vi "P2019 TB INCAR_Run Auto.vi"(7 "ModuloIN":u32=10, 8 "error in (no error)":errorcluster, 9 "Comunicaciones":T7={"Flujo_1"="ASRL6::INSTR", "Brk1"=FALSE, "Flujo_2"="ASRL6::INSTR", "Brk2"=FALSE, "Flujo_3"="ASRL6::INSTR", "Brk3"=FALSE, "Flujo_4"="ASRL6::INSTR", "Brk4"=FALSE, "Eurothe"="ASRL6::INSTR", "Eurot"=FALSE, "Balanza"="ASRL6::INSTR", "Bal"=FALSE, "eValPos"="ASRL6::INSTR", "eVal"=FALSE, "flowbus"="ASRL6::INSTR", "fb"=FALSE}, 10 "Secuencia":string[](array[string])) -> (0 "error out":errorcluster)   [LabVIEW 2013]
uses:
  Controles/P2022 Datos Control.ctl
  Controles/P2018 Com Control.ctl
  modbusEurotherm P116_485/4xP116.ctl
  Controles/P2018 DisbalTB Control.ctl
  Controles/P2018 Arduino Control.ctl
  Controles/P2018 Bronkhorst Control.ctl
  serialBronkhorst/_s_TablaBronkhorst.ctl
  modbusEurotherm P116_485/P2018 Eurotherm Control.ctl
  Controles/Data Type.ctl
  Display/Display_Command Control.ctl
  Controles/P2018 runAuto Control.ctl
  File/File_Module Control.ctl
  Timing/Timing_Module Control.ctl
  modbusEurotherm P116_485/Eurotherm_Hardware_Module Control.ctl
  serialTermobDisbal/Multicard III_Hardware_Module Control.ctl
  P2022 TB INCAR GLOBALES.vi
panel:
  out "Valvula":bool=TRUE
  out "TIEMPO (m)":dbl
  out "EURO_P116":T1
  out "BRONKHORST":T3={"Dispositivos"=[["3", "NO", "M0000013", "Air", "10", "ln/mn", "0", "0"], ["4", "NO", "M0000014", "Air", "10", "ln/mn", "0", "0"], ["5", "NO", "M0000015", "Air", "10", "ln/mn", "0", "0"], ["6", "NO", "M0000016", "Air", "10", "ln/mn", "0", "0"], ["7", "NO", "M0000017", "Air", "10", "ln/mn", "0", "0"], ["8", "NO", "M0000018", "Air", "10", "ln/mn", "0", "0"]], "NuevosSP"=[["0", "NO", "M0000013", "Air", "1", "ln/mn", "0", "0"], ["0", "NO", "M0000014", "Air", "1", "ln/mn", "0", "0"], ["0", "NO", "M0000015", "Air", "1", "ln/mn", "0", "0"], ["0", "NO", "M0000016", "Air", "1", "ln/mn", "0", "0"], ["0", "NO", "M0000017", "Air", "1", "ln/mn", "0", "0"], ["0", "NO", "M0000018", "Air", "1", "ln/mn", "0", "0"]], "Nodes"=8, "Delay(s)"=0.075}
  out "ARDUINO":T5
  out "DISBAL":T6 caption="tarjetaPresion"
  out "RateSP":T2
  out "NuevoSP":T2
  out "Modulo":u32
  out "Timestring":string
  out "MedidaModulo":u32
  out "Max_t(s)":dbl format="%.1f"
  out "Delta t(s)":dbl format="%.1f"
  out "Delta T(C)":dbl format="%.1f"
  out "TStable":bool
  out "Datos":T8 {"fFSET4" format="%.2g"; "fFSET3" format="%.2g"; "fFSET2" format="%.2g"; "fFSET1" format="%.2g"; "fFLUJO4" format="%.2g"; "fFLUJO2" format="%.2g"; "fFLUJO1" format="%.2g"; "fFLUJO3" format="%.2g"; "T_EXTRA" format="%.2g"; "TSET_EXTRA" format="%.2g"; "T_CINTA" format="%.2g"; "TSET_CINTA" format="%.2g"; "sFSET4" format="%.2g"; "POSICION" format="%.2g"; "TEMP_SUP" format="%.2g"; "TSET_SUP" format="%.2g"; "PESO_TB" format="%.2g"; "TEMP_TB" format="%.2g"; "TEMP_INF" format="%.2g"; "sFSET3" format="%.2g"; "sFSET2" format="%.2g"; "sFSET1" format="%.2g"; "V_VAPOR" format="%.2g"; "sFLUJO4" format="%.2g"; "sFLUJO2" format="%.2g"; "sFLUJO1" format="%.2g"; "TSET_INF" format="%.2g"; "TIEMPO" format="%.2g"; "sFLUJO3" format="%.2g"}
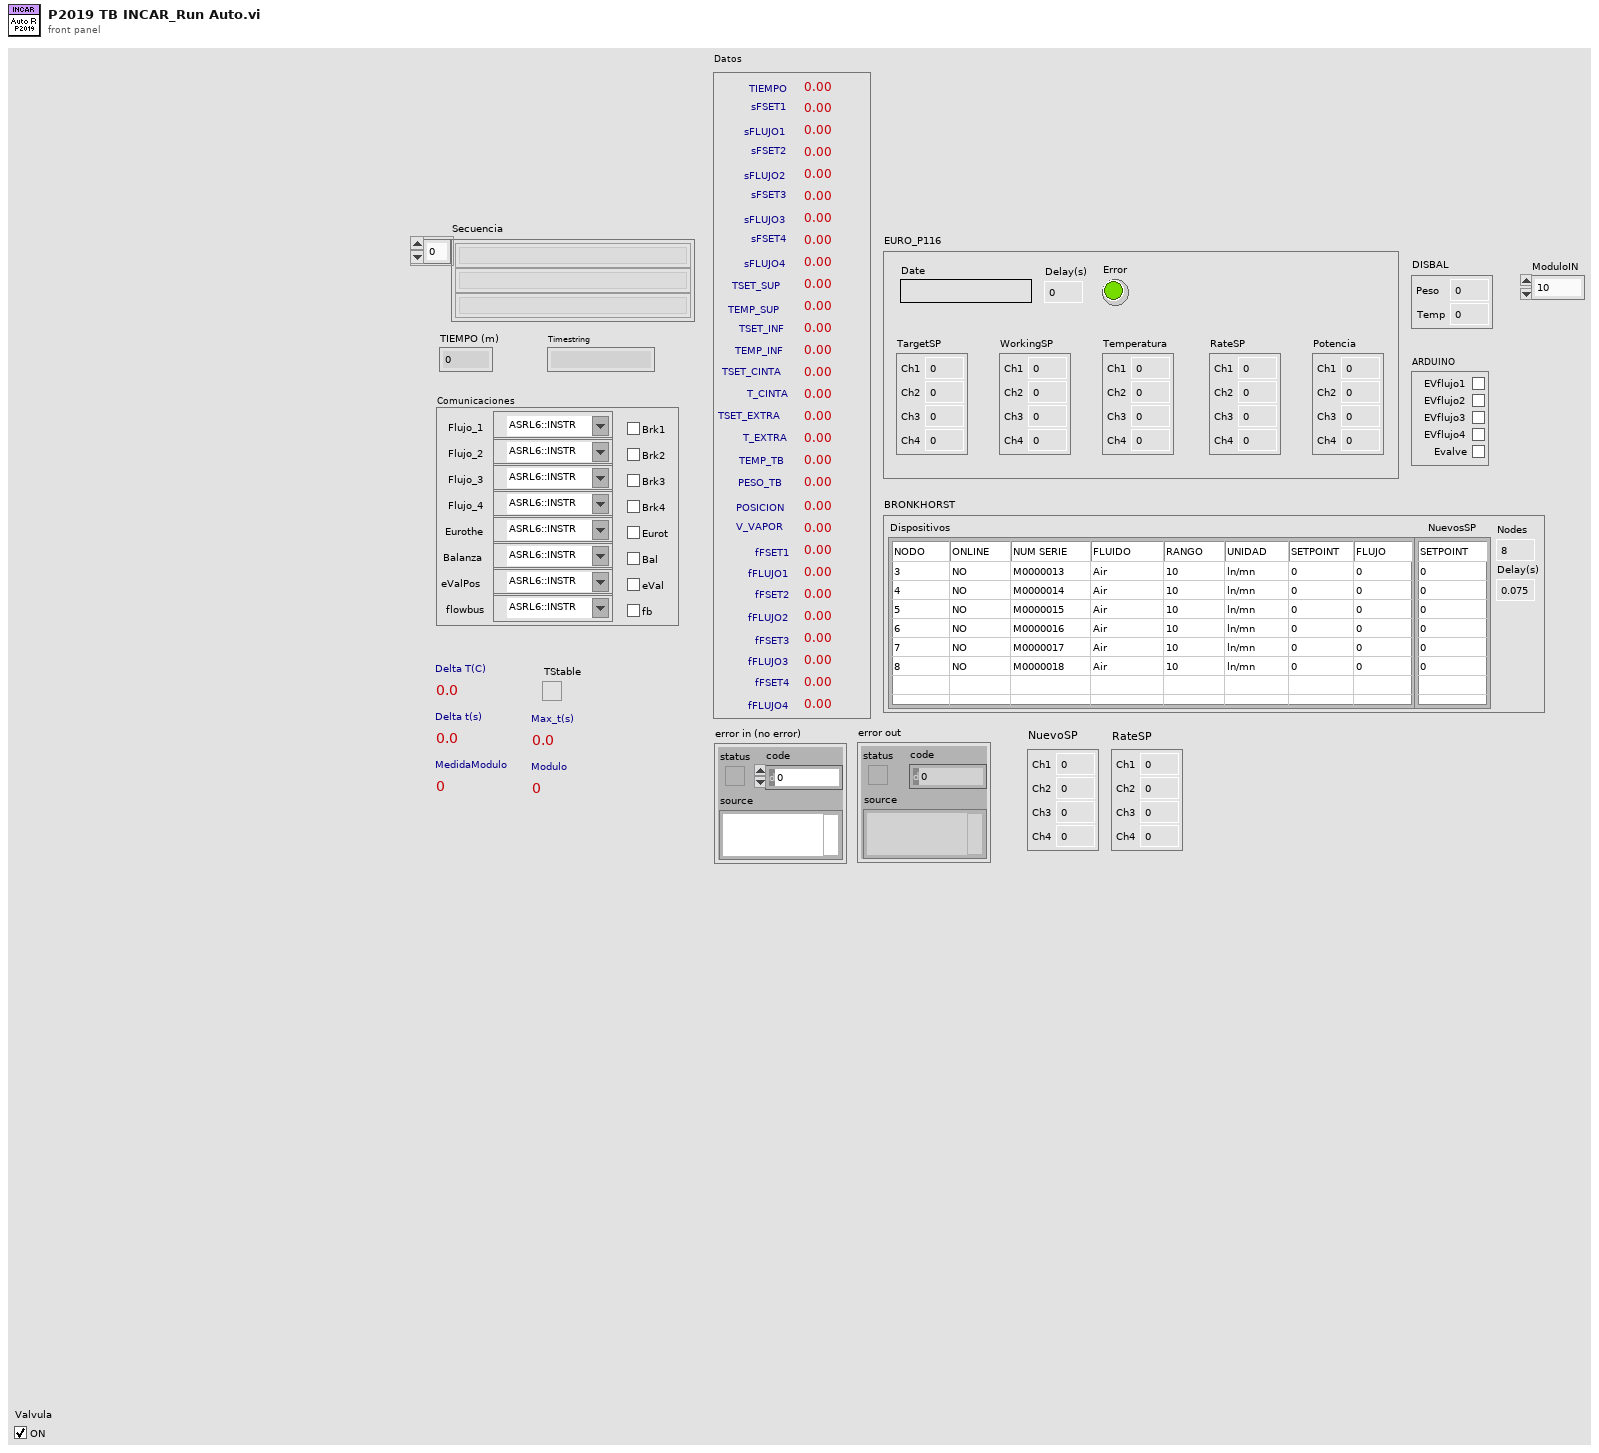
[diagram p1: front panel]
types:
  T1 = typedef "P2018 Eurotherm Control.ctl" = cluster{"TargetSP":T2, "WorkingSP":T2, "Temperatura":T2, "Error":bool, "Date":string, "Delay(s)":dbl, "RateSP":T2, "Potencia":T2}
  T2 = typedef "4xP116.ctl" = cluster{"Ch1":dbl, "Ch2":dbl, "Ch3":dbl, "Ch4":dbl}
  T3 = typedef "P2018 Bronkhorst Control.ctl" = cluster{"Dispositivos":T4, "NuevosSP":string[][], "Nodes":u32, "Delay(s)":dbl}
  T4 = typedef "_s_TablaBronkhorst.ctl" = string[][]
  T5 = typedef "P2018 Arduino Control.ctl" = cluster{"EVflujo1":bool, "EVflujo2":bool, "EVflujo3":bool, "EVflujo4":bool, "Evalve":bool}
  T6 = typedef "P2018 DisbalTB Control.ctl" = cluster{"Peso":dbl, "Temp":dbl}
  T7 = typedef "P2018 Com Control.ctl" = cluster{"Flujo_1":refnum<visa-resource-name>, "Brk1":bool, "Flujo_2":refnum<visa-resource-name>, "Brk2":bool, "Flujo_3":refnum<visa-resource-name>, "Brk3":bool, "Flujo_4":refnum<visa-resource-name>, "Brk4":bool, "Eurothe":refnum<visa-resource-name>, "Eurot":bool, "Balanza":refnum<visa-resource-name>, "Bal":bool, "eValPos":refnum<visa-resource-name>, "eVal":bool, "flowbus":refnum<visa-resource-name>, "fb":bool}
  T8 = typedef "P2022 Datos Control.ctl" = cluster{"TIEMPO":dbl, "sFSET1":dbl, "sFLUJO1":dbl, "sFSET2":dbl, "sFLUJO2":dbl, "sFSET3":dbl, "sFLUJO3":dbl, "sFSET4":dbl, "sFLUJO4":dbl, "TSET_SUP":dbl, "TEMP_SUP":dbl, "TSET_INF":dbl, "TEMP_INF":dbl, "TSET_CINTA":dbl, "T_CINTA":dbl, "TSET_EXTRA":dbl, "T_EXTRA":dbl, "TEMP_TB":dbl, "PESO_TB":dbl, "POSICION":dbl, "V_VAPOR":dbl, "fFSET1":dbl, "fFLUJO1":dbl, "fFSET2":dbl, "fFLUJO2":dbl, "fFSET3":dbl, "fFLUJO3":dbl, "fFSET4":dbl, "fFLUJO4":dbl}
  T9 = typedef "Data Type.ctl" = enum16{"Init FP", "En/Dis FP Ctls", "Update FP", "Upd Status", "Upd Seq"}
  T10 = typedef "Display_Command Control.ctl" = enum16{"Initialize", "Generate Event", "Shutdown"}
  T11 = typedef "P2018 runAuto Control.ctl" = enum16{"inicializar", "testComando", "cambioGasesS", "cambioGasesF", "cambioValvulas", "cambioTemperaturas", "cEstableTemp?", "cReadTiempo", "cReadGases", "cReadTemperaturas", "cReadTermobalanza", "cSaveDatos", "cWait", "cambioTiempos", "tAgotadoTiempo?", "tReadTiempo", "tReadGases", "tReadTemperaturas", "tReadTermobalanza", "tSaveDatos", "tWait", "finalizar"}
  T12 = typedef "File_Module Control.ctl" = enum16{"Initialize", "Save Head", "Save Data", "Shutdown"}
  T13 = typedef "Eurotherm_Hardware_Module Control.ctl" = enum16{"Initialize", "Write SP", "Read SP+PV", "Write Rate", "Set P", "Set I", "Set D", "Shutdown"}
  T14 = typedef "Timing_Module Control.ctl" = enum16{"Initialize Time", "Check Time"}
  T15 = typedef "Multicard III_Hardware_Module Control.ctl" = enum16{"Initialize", "Cero", "Span", "Read ugr", "Read mgr", "Read A/D", "Read T", "Number readings", "Thermocouple type", "Status", "Shutdown"}
  T16 = typedef "P2019 SetpointsFlows.ctl" = cluster{"SP1":dbl, "SP2":dbl, "SP3":dbl, "SP4":dbl}
  T17 = typedef "_f_TablaBronkhorst.ctl" = string[][]
  T18 = enum16{"Add 1", "Add 2", "Add 10", "Add 11", "Add 12", "Add 13"}[]
  T19 = cluster{"processVal":dbl, "targetSP":dbl, "workingSP":dbl, "workingOut":dbl}
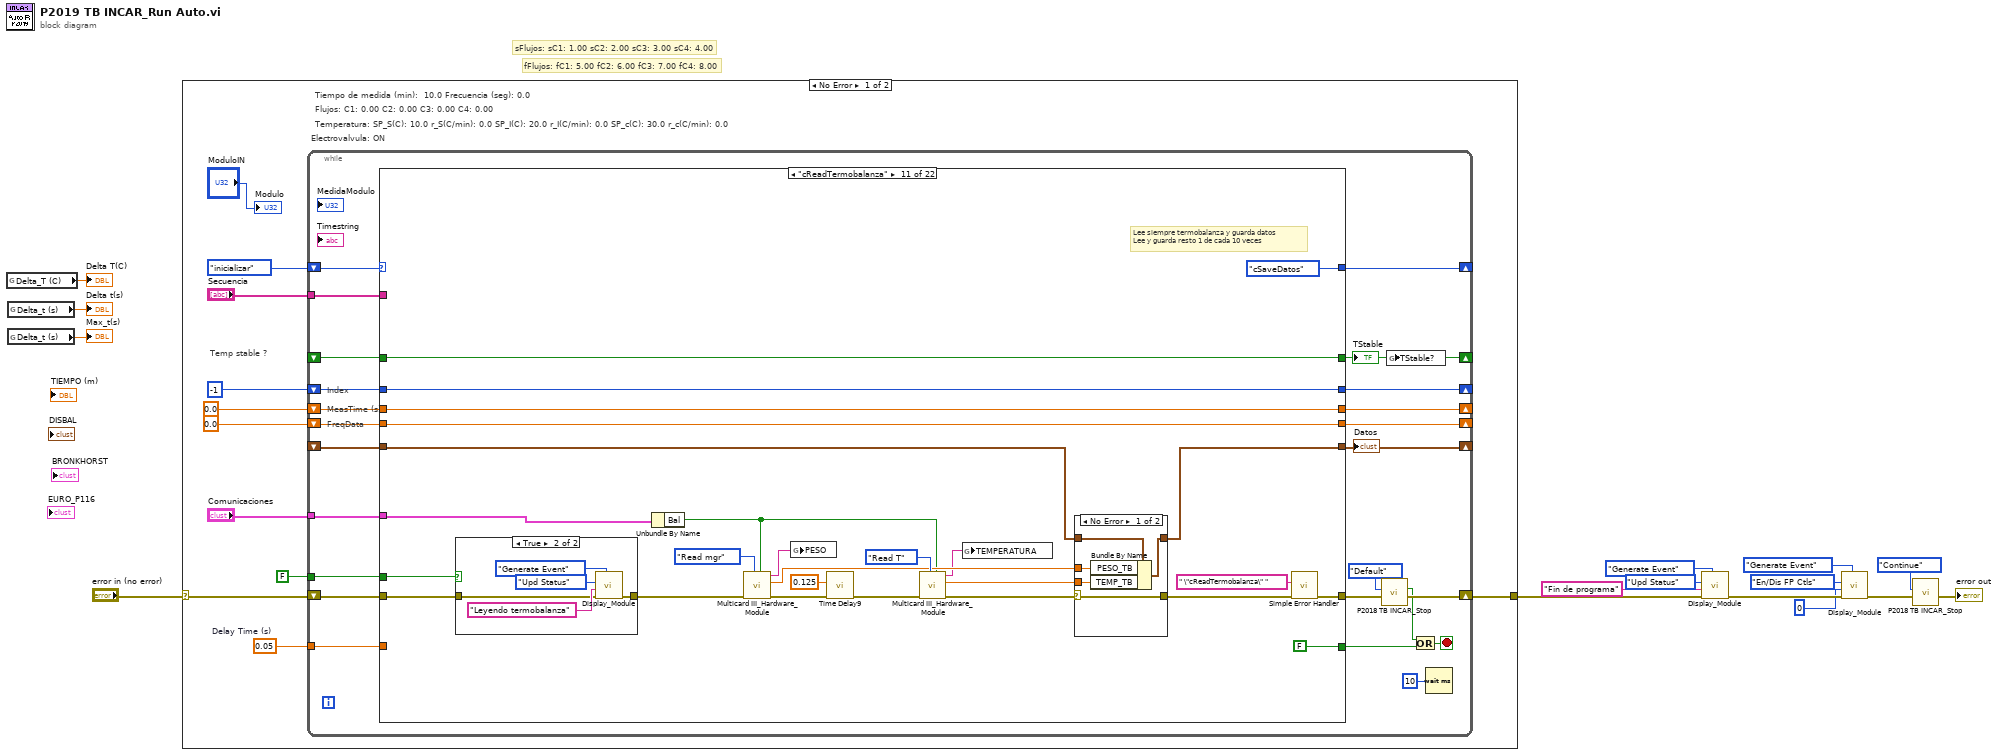
[diagram p0: block diagram]
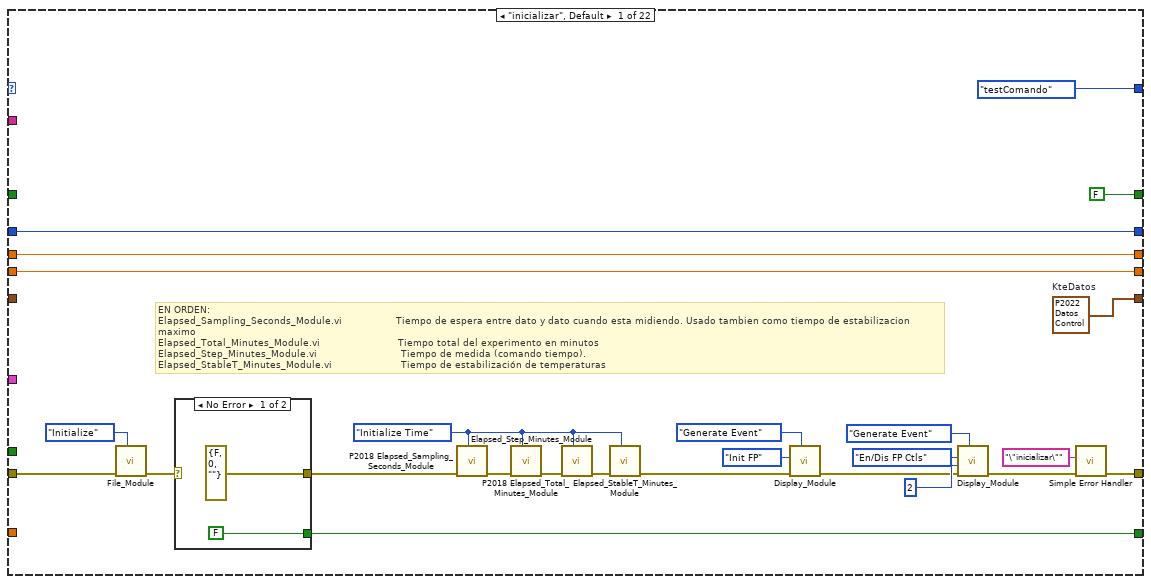
[diagram p2: hidden frame]
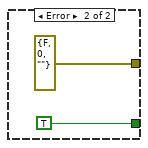
[diagram p3: hidden frame]
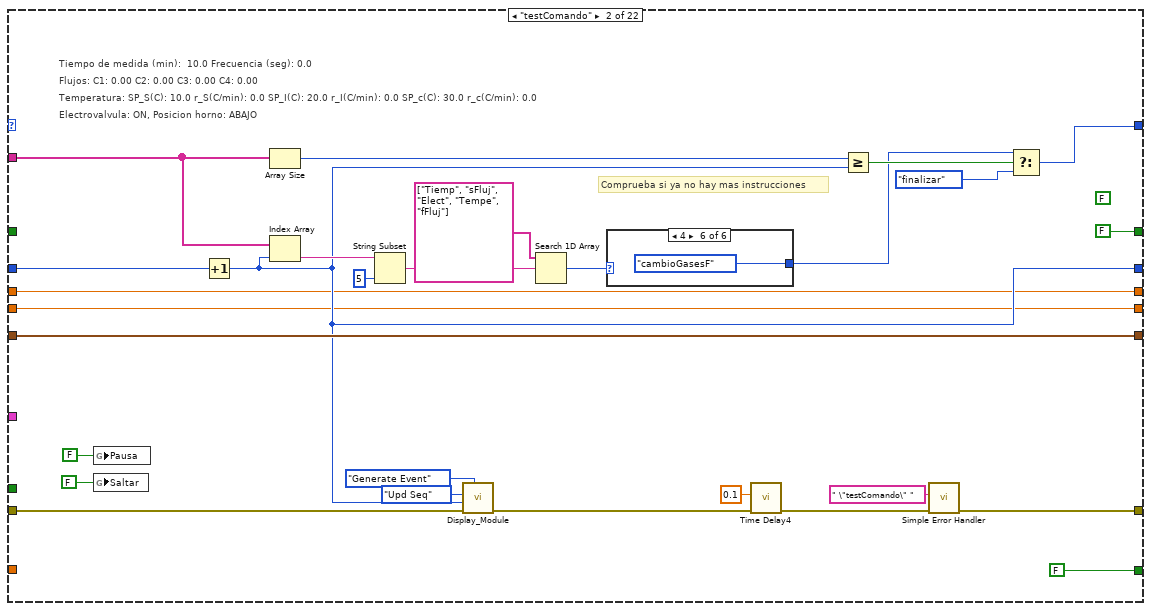
[diagram p4: hidden frame]
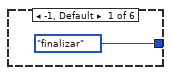
[diagram p5: hidden frame]
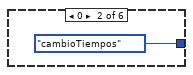
[diagram p6: hidden frame]
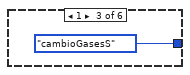
[diagram p7: hidden frame]
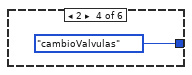
[diagram p8: hidden frame]
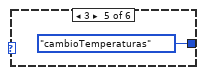
[diagram p9: hidden frame]
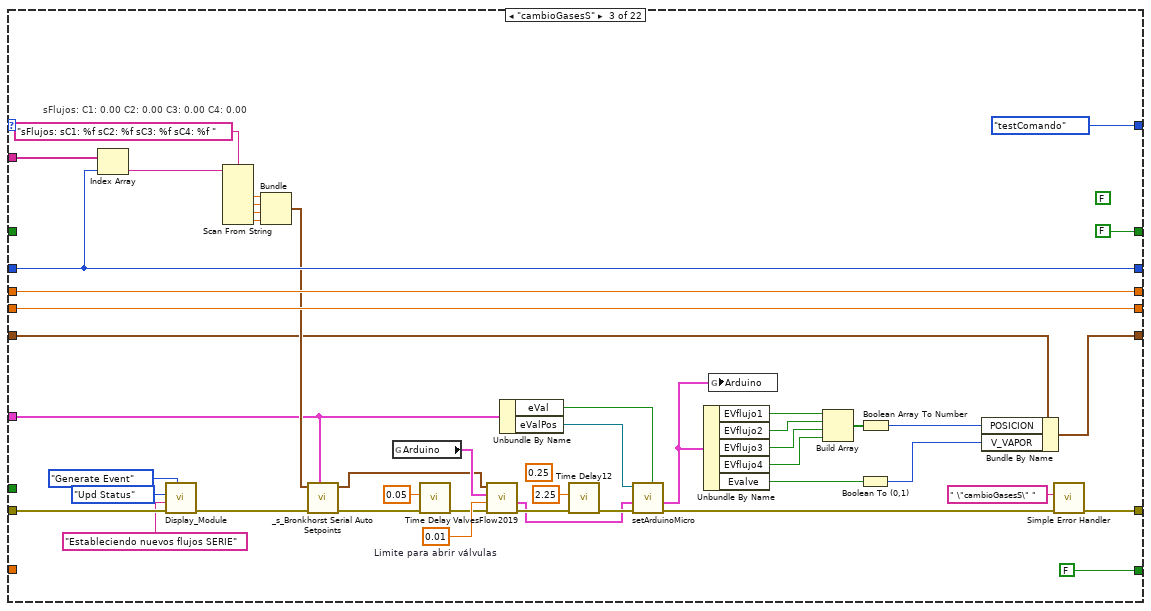
[diagram p10: hidden frame]
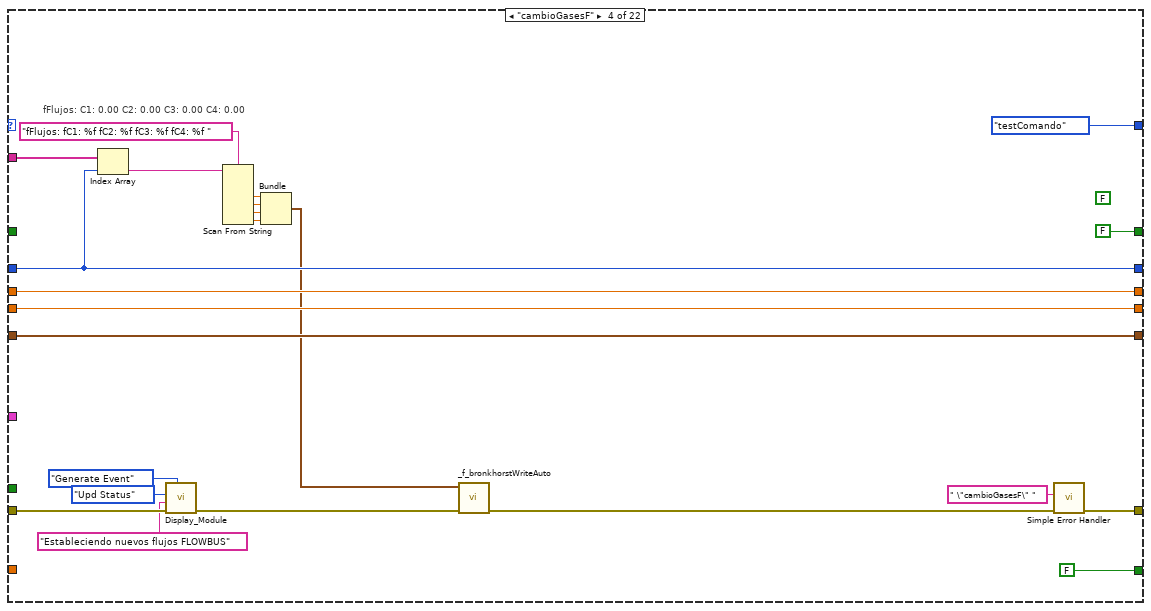
[diagram p11: hidden frame]
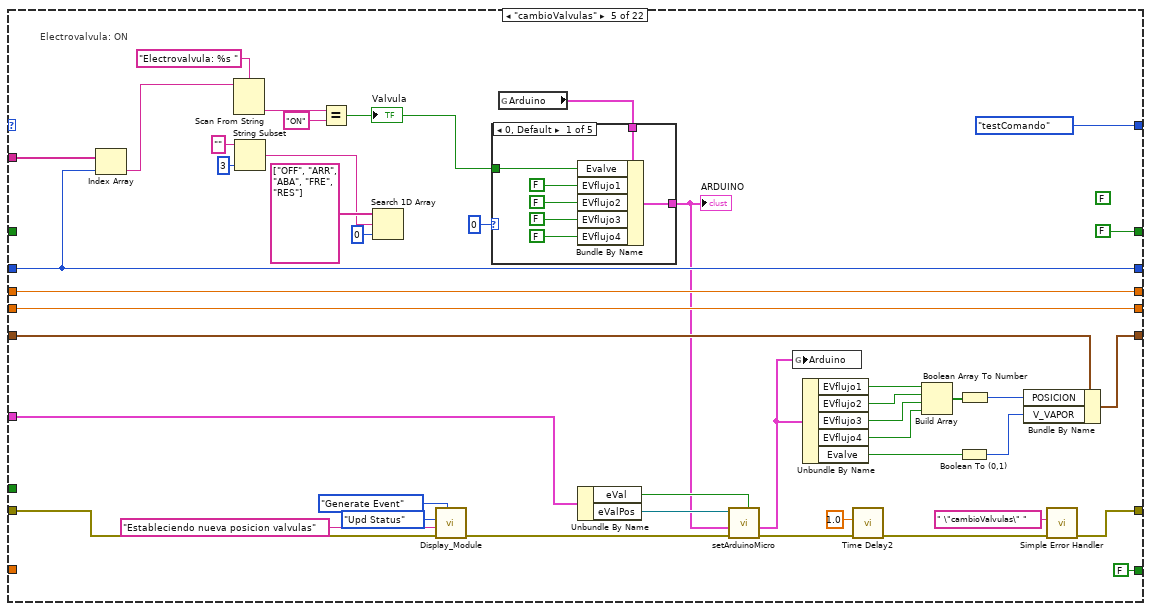
[diagram p12: hidden frame]
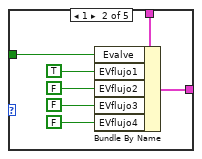
[diagram p13: hidden frame]
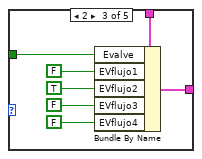
[diagram p14: hidden frame]
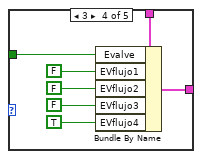
[diagram p15: hidden frame]
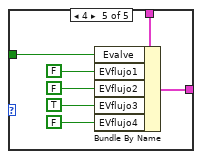
[diagram p16: hidden frame]
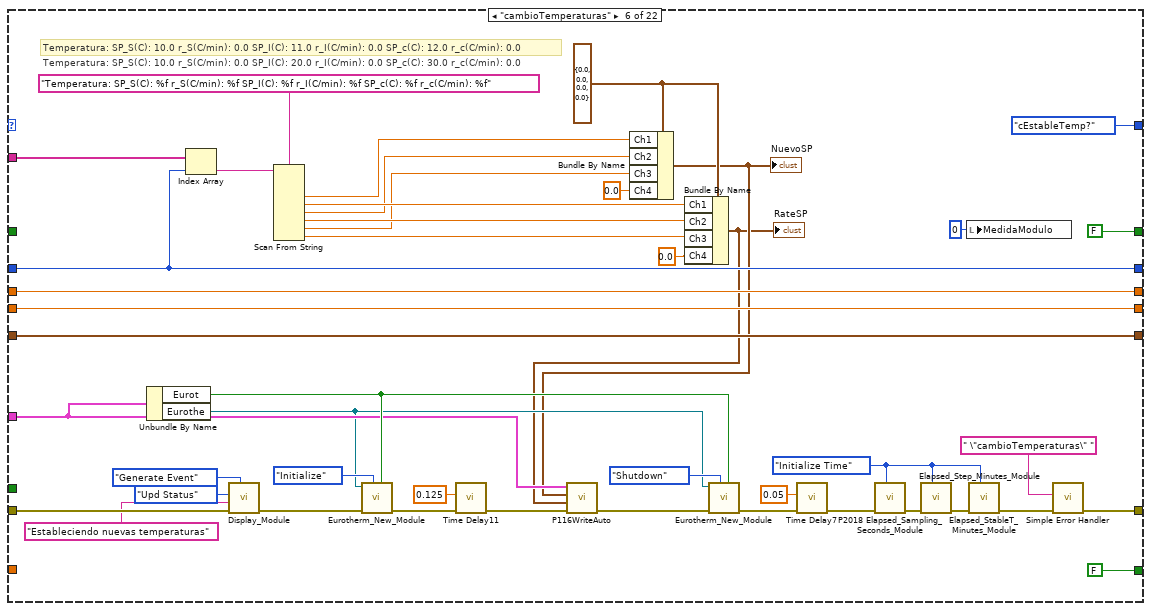
[diagram p17: hidden frame]
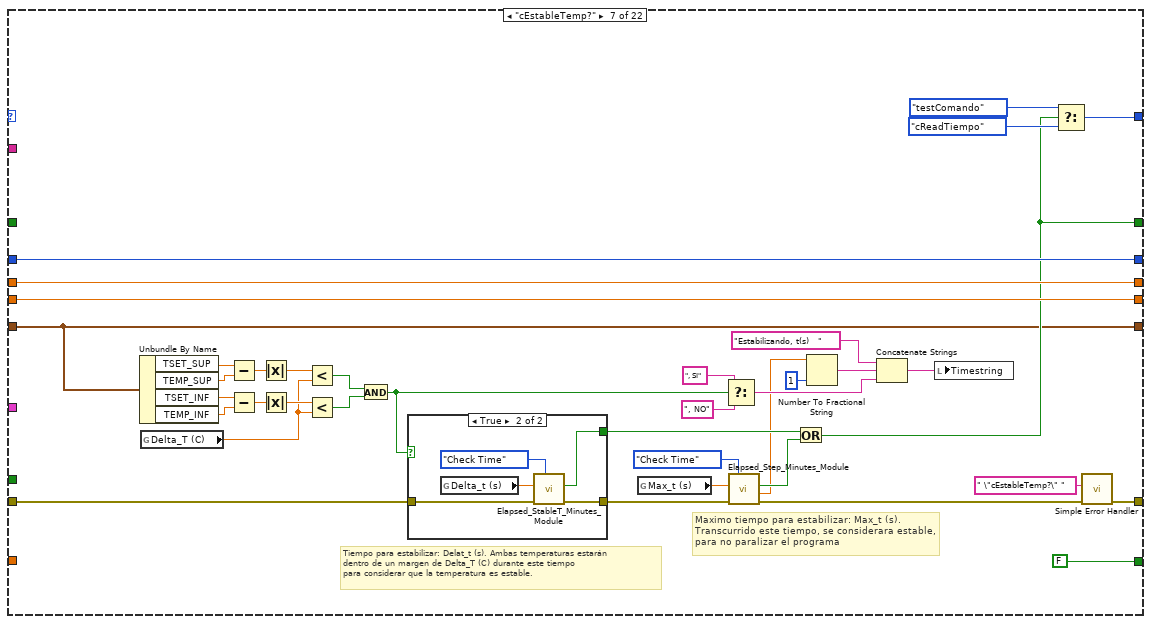
[diagram p18: hidden frame]
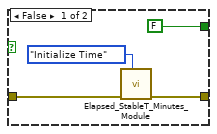
[diagram p19: hidden frame]
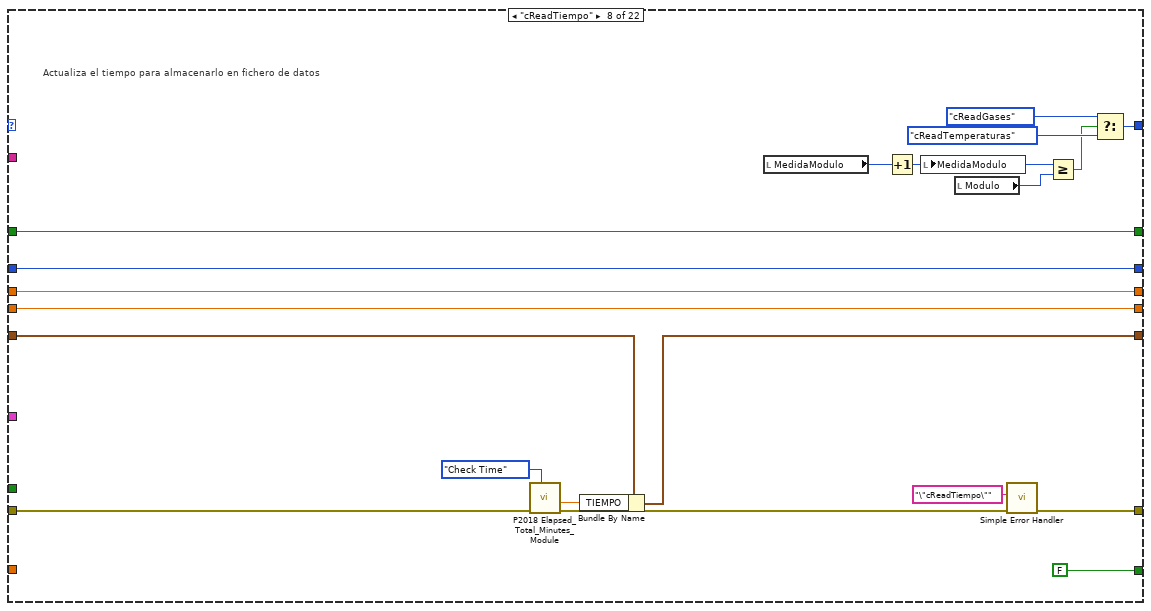
[diagram p20: hidden frame]
diagram:
  # "fFlujos: fC1: 5.00 fC2: 6.00 fC3: 7.00 fC4: 8.00"
  # "sFlujos: sC1: 1.00 sC2: 2.00 sC3: 3.00 sC4: 4.00"
  n1 = global read "P2022 TB INCAR GLOBALES.vi" "Delta_T (C)"() -> (→"Delta T(C)":dbl)
  n2 = global read "P2022 TB INCAR GLOBALES.vi" "Delta_t (s)"() -> (→"Delta t(s)":dbl)
  n3 = global read "P2022 TB INCAR GLOBALES.vi" "Delta_t (s)"() -> (→"Max_t(s)":dbl)
  n4 = case shown="No Error" "error in (no error)" {
    selector: "error in (no error)" -> [w26 w866]
    tunnel: [w25 w866] -> w7
    frame No Error {
      w17 = 0.05  # Delay Time (s)
      # "Electrovalvula: ON"
      # "Flujos: C1: 0.00 C2: 0.00 C3: 0.00 C4: 0.00"
      # "Tiempo de medida (min):  10.0 Frecuencia (seg): 0.0"
      # "Temperatura: SP_S(C): 10.0 r_S(C/min): 0.0 SP_I(C): 20.0 r_I(C/min): 0.0 SP_c(C): 30.0 r_c(C/min): 0.0"
      # "Temp stable ?"
      n5 = while {
        shift-right: [w41] -> _
        shift-left: P2018_runAuto_Control."inicializar" ("Command") -> [w46]
        shift-right: [w45] -> w25
        shift-left: w26 -> [w47]
        shift-right: [w32] -> _
        shift-left: _ -> [w40]
        tunnel: "Secuencia" -> [w39]
        shift-right: [w37] -> _
        shift-left: -1 ("milliseconds to wait") -> [w38]
        shift-right: [w34] -> _
        shift-left: 0.0 -> [w35]
        shift-right: [w33] -> _
        shift-left: 0.0 -> [w36]
        tunnel: "Comunicaciones" -> [w31]
        shift-right: [w29] -> _
        shift-left: _ -> [w30]
        tunnel: w17 -> [w28]
        tunnel: FALSE -> [w27]
        stop <- w49 stop-if-true
        # "FreqData"
        # "Index"
        # "MeasTime (s)"
        n6 = case shown="\"cReadTermobalanza\"" w46 {
          tunnel: [w60 FALSE FALSE FALSE FALSE FALSE FALSE FALSE FALSE FALSE FALSE FALSE FALSE FALSE FALSE FALSE FALSE FALSE FALSE FALSE FALSE TRUE] -> w48
          tunnel: w47 -> [w74 w88 w157 w180 w224 w304 w307 w367 w419 w445 w501 w540 w561 w582 w615 w639 w678 w708 w773 w812 w835 w859]
          tunnel: [w55 w82 w139 w166 w211 w288 w311 w362 w414 w456 w493 w527 w545 w578 w597 w634 w689 w728 w765 w799 w815 w848] -> w44
          tunnel: [P2018_runAuto_Control."testComando" ("Command") w101 P2018_runAuto_Control."testComando" ("Command") P2018_runAuto_Control."testComando" ("Command") P2018_runAuto_Control."testComando" ("Command") P2018_runAuto_Control."cEstableTemp?" ("Command") w338 w357 P2018_runAuto_Control."cReadTemperaturas" ("Command") P2018_runAuto_Control."cReadTermobalanza" ("Command") P2018_runAuto_Control."cSaveDatos" ("Command") P2018_runAuto_Control."cWait" ("Command") w564 P2018_runAuto_Control."tAgotadoTiempo?" ("Command") w618 w630 P2018_runAuto_Control."tReadTemperaturas" ("Command") P2018_runAuto_Control."tReadTermobalanza" ("Command") P2018_runAuto_Control."tSaveDatos" ("Command") P2018_runAuto_Control."tWait" ("Command") w838 P2018_runAuto_Control."finalizar" ("Command")] -> w41
          tunnel: [w72 w106 w114 w163 w214 w299 w313 w370 w374 w442 w500 w531 w563 w588 w617 w642 w646 w705 w772 w803 w837 w863] -> w32
          tunnel: w40 -> [_ w106 w115 w163 w215 w299 w313 w373 w418 w441 w499 w531 w563 w588 w617 w645 w677 w704 w771 w803 w837 w863]
          tunnel: w39 -> [_ w104 w159 w182 w226 w306 _ _ _ _ _ _ _ w591 _ _ _ _ _ _ _ _]
          tunnel: w38 -> [w68 w94 w155 w178 w222 w302 w341 w371 w422 w460 w511 w537 w552 w589 w609 w643 w694 w732 w783 w809 w826 w862]
          tunnel: [w68 w92 w155 w178 w222 w302 w341 w371 w422 w460 w511 w537 w552 w589 w609 w643 w694 w732 w783 w809 w826 w862] -> w37
          tunnel: w36 -> [w66 w89 w144 w167 w217 w294 w342 w368 w420 w458 w509 w535 w542 _ w605 w640 w692 w730 w781 w807 w814 w852]
          tunnel: w35 -> [w67 w90 w145 w168 w218 w295 w343 w369 w421 w459 w510 w536 w551 _ w601 w641 w693 w731 w782 w808 w825 w853]
          tunnel: [w67 w90 w145 w168 w218 w295 w343 w369 w421 w459 w510 w536 w551 w583 w601 w641 w693 w731 w782 w808 w825 w853] -> w34
          tunnel: [w66 w89 w144 w167 w217 w294 w342 w368 w420 w458 w509 w535 w542 w590 w605 w640 w692 w730 w781 w807 w814 w852] -> w33
          tunnel: w31 -> [_ _ w122 _ w186 w277 _ _ w412 w444 w502 _ _ _ _ _ w679 w706 w774 _ _ _]
          tunnel: w30 -> [_ _ _ _ _ _ _ w365 w416 _ w495 w530 w548 w580 w599 w637 w691 w726 w767 w802 w818 w851]
          tunnel: [FALSE ("TStable?") FALSE ("TStable?") FALSE ("TStable?") FALSE ("TStable?") FALSE ("TStable?") FALSE ("TStable?") w316 w365 w416 FALSE ("TStable?") w495 w530 w548 w580 w599 w637 w691 w726 w767 w802 w818 w851] -> w29
          tunnel: w28 -> [_ _ _ _ _ _ _ _ w404 _ _ _ _ _ _ _ w676 _ _ _ _ _]
          tunnel: w27 -> [_ _ _ _ _ _ _ _ w403 w431 w489 _ _ _ _ _ w675 w703 w761 _ _ _]
          frame "inicializar", Default {
            w51 = Timing_Module_Control."Initialize Time" ("Command")
            w72 = T8 {"TIEMPO"=0.0, "sFSET1"=0.0, "sFLUJO1"=0.0, "sFSET2"=0.0, "sFLUJO2"=0.0, "sFSET3"=0.0, "sFLUJO3"=0.0, "sFSET4"=0.0, "sFLUJO4"=0.0, "TSET_SUP"=0.0, "TEMP_SUP"=0.0, "TSET_INF"=0.0, "TEMP_INF"=0.0, "TSET_CINTA"=0.0, "T_CINTA"=0.0, "TSET_EXTRA"=0.0, "T_EXTRA"=0.0, "TEMP_TB"=0.0, "PESO_TB"=0.0, "POSICION"=0.0, "V_VAPOR"=0.0, "fFSET1"=0.0, "fFLUJO1"=0.0, "fFSET2"=0.0, "fFLUJO2"=0.0, "fFSET3"=0.0, "fFLUJO3"=0.0, "fFSET4"=0.0, "fFLUJO4"=0.0}  # KteDatos
            # "EN ORDEN:\nElapsed_Sampling_Seconds_Module.vi                  Tiempo de espera entre dato y dato cuando esta midiendo. Usado tambien como tiempo de estabilizacion maximo \nElapsed_Total_Minutes_Module.vi                          Tiempo total del experimento en minutos\nElapsed_Step_Minutes_Module.vi                            Tiempo de medida (comando tiempo). \nElapsed_StableT_Minutes_Module.vi                       Tiempo de estabilización de temperaturas"
            n7 = call "File_Module.vi"("Command"=File_Module_Control."Initialize", "error in (no error)"=w74) -> ("error out"=w62:errorcluster)  [unwired: 8 in, 1 out]
            n8 = case shown="No Error" w62 {
              tunnel: [errorcluster {"status"=FALSE, "code"=0, "source"=""} ("error out") errorcluster {"status"=FALSE, "code"=0, "source"=""} ("error out")] -> w61
              tunnel: [FALSE TRUE] -> w60
              frame No Error {
              }
              frame Error {
              }
            }
            n9 = call "P2018 Elapsed_Sampling_Seconds_Module.vi"("Command"=w51, "error in (no error)"=w61) -> ("error out"=w59:errorcluster)  [unwired: 7 in, 2 out]
            n10 = call "P2018 Elapsed_Total_Minutes_Module.vi"("Command"=w51, "error in (no error)"=w59) -> ("error out"=w58:errorcluster)  [unwired: 7 in, 2 out]
            n11 = call "Elapsed_Step_Minutes_Module.vi"("Command"=w51, "error in (no error)"=w58) -> ("error out"=w53:errorcluster)  [unwired: 7 in, 2 out]
            n12 = call "Elapsed_StableT_Minutes_Module.vi"("Command"=w51, "error in (no error)"=w53) -> ("error out"=w52:errorcluster)  [unwired: 7 in, 2 out]
            n13 = call "Display_Module.vi"("Command"=Display_Command_Control."Generate Event", "error in (no error)"=w52, "Data Type"=Data_Type."Init FP") -> ("error out"=w63:errorcluster)  [unwired: 8 in]
            n14 = call "Display_Module.vi"("Command"=Display_Command_Control."Generate Event", "error in (no error)"=w63, "Data"=2, "Data Type"=Data_Type."En/Dis FP Ctls") -> ("error out"=w56:errorcluster)  [unwired: 7 in]
            n15 = call <vilib>:"Simple Error Handler.vi"("error source (\" \")"="\"inicializar\"" ("error source (\" \")"), "error in (no error)"=w56) -> ("error out"=w55:errorcluster)  [unwired: 3 in, 4 out]
          }
          frame "testComando" {
            (unwired) FALSE ("TStable?")
            # "Electrovalvula: ON, Posicion horno: ABAJO"
            # "Flujos: C1: 0.00 C2: 0.00 C3: 0.00 C4: 0.00"
            # "Tiempo de medida (min):  10.0 Frecuencia (seg): 0.0"
            # "Temperatura: SP_S(C): 10.0 r_S(C/min): 0.0 SP_I(C): 20.0 r_I(C/min): 0.0 SP_c(C): 30.0 r_c(C/min): 0.0"
            # "Comprueba si ya no hay mas instrucciones"
            n16 = global write "P2022 TB INCAR GLOBALES.vi" "Pausa"(FALSE ("Saltar")) -> ()
            n17 = global write "P2022 TB INCAR GLOBALES.vi" "Saltar"(FALSE ("Saltar")) -> ()
            n18 = Increment(x=w94) -> (x+1=w92:i32)
            n19 = Array Size(array=w104) -> (size(s)=w103:i32)
            n20 = Index Array(array=w104, index=w92) -> (element=w99:string)
            n21 = String Subset(string=w99, length (rest)=5 ("length (rest)")) -> (substring=w97:string)  [unwired: 1 in]
            n22 = call "Display_Module.vi"("Command"=Display_Command_Control."Generate Event", "error in (no error)"=w88, "Data"=w92, "Data Type"=Data_Type."Upd Seq") -> ("error out"=w85:errorcluster)  [unwired: 7 in]
            n23 = Search 1D Array(1D array=string[] ["Tiemp", "sFluj", "Elect", "Tempe", "fFluj"], element=w97) -> (index of element=w96:i32)  [unwired: 1 in]
            n24 = case shown="4" w96 {
              tunnel: [P2018_runAuto_Control."finalizar" ("Command") P2018_runAuto_Control."cambioTiempos" ("Command") P2018_runAuto_Control."cambioGasesS" ("Command") P2018_runAuto_Control."cambioValvulas" ("Command") P2018_runAuto_Control."cambioTemperaturas" ("Command") P2018_runAuto_Control."cambioGasesF" ("Command")] -> w95
              frame -1, Default {
              }
              frame 0 {
              }
              frame 1 {
              }
              frame 2 {
              }
              frame 3 {
              }
              frame 4 {
              }
            }
            n25 = call "Time Delay4"("error in (no error)"=w85, "Delay Time (s)"=0.1) -> ("error out"=w83:errorcluster)  [unwired: 9 in]
            n26 = Greater Or Equal?(x=w103, y=w92) -> (x >= y?=w102:bool)
            n27 = call <vilib>:"Simple Error Handler.vi"("error source (\" \")"=" \"testComando\" " ("error source (\" \")"), "error in (no error)"=w83) -> ("error out"=w82:errorcluster)  [unwired: 3 in, 4 out]
            n28 = Select(t=w95, s=w102, f=P2018_runAuto_Control."finalizar" ("Command")) -> (s? t:f=w101:T11)
          }
          frame "cambioGasesS" {
            (unwired) 0.25 ("Delay Time (s)")
            w123 = 0.01  # Limite para abrir válvulas
            (unwired) FALSE ("TStable?")
            # "sFlujos: C1: 0.00 C2: 0.00 C3: 0.00 C4: 0.00"
            n29 = Index Array(array=w159, index=w155) -> (element=w146:string)
            n30 = call "Display_Module.vi"("Command"=Display_Command_Control."Generate Event", "error in (no error)"=w157, "Data"="Estableciendo nuevos flujos SERIE" ("element"), "Data Type"=Data_Type."Upd Status") -> ("error out"=w142:errorcluster)  [unwired: 7 in]
            n31 = Scan From String(format string="sFlujos: sC1: %f sC2: %f sC3: %f sC4: %f ", input string=w146) -> (output 1=w150:dbl, output 2=w149:dbl, output 3=w148:dbl, output 4=w147:dbl)  [unwired: 6 in, 3 out]
            n32 = Bundle(w150, w149, w148, w147) -> (w140:cluster{dbl, dbl, dbl, dbl})  [unwired: 1 in]
            n33 = call "_s_Bronkhorst Serial Auto Setpoints.vi"("Comunicaciones"=w122, "error in (no error)"=w142, "Datos"=w140) -> ("error out"=w141:errorcluster, "Setpoints"=w116:T16)  [unwired: 7 in]
            n34 = global read "P2022 TB INCAR GLOBALES.vi" "Arduino"() -> (w121:T5)
            n35 = call "Time Delay"("error in (no error)"=w141, "Delay Time (s)"=0.05) -> ("error out"=w120:errorcluster)  [unwired: 9 in]
            n36 = call "ValvesFlow2019.vi"("error in (no error)"=w120, "Limite"=w123, "ESTADO in"=w121, "Setpoints"=w116) -> ("error out"=w135:errorcluster, "ESTADO out"=w117:T5)  [unwired: 4 in]
            n37 = Unbundle By Name(w122) -> ("eVal"=w125:bool, "eValPos"=w124:refnum<visa-resource-name>)
            n38 = call "Time Delay12"("error in (no error)"=w135, "Delay Time (s)"=2.25) -> ("error out"=w136:errorcluster)  [unwired: 9 in]
            n39 = call "setArduinoMicro.vi"("Enable"=w125, "error in"=w136, "ESTADO"=w117, "VISA resource name"=w124) -> ("error out"=w119:errorcluster, "ESTADO 2"=w118:T5)  [unwired: 6 in]
            n40 = Unbundle By Name(w118) -> ("EVflujo1"=w127:bool, "EVflujo2"=w128:bool, "EVflujo3"=w129:bool, "EVflujo4"=w130:bool, "Evalve"=w126:bool)
            n41 = global write "P2022 TB INCAR GLOBALES.vi" "Arduino"(w118) -> ()
            n42 = Build Array(w127, w128, w129, w130) -> (w131:bool[])
            n43 = Boolean To (0,1)(Boolean=w126) -> (0, 1=w133:i16)
            n44 = Boolean Array To Number(Boolean array=w131) -> (number=w132:u32)
            n45 = Bundle By Name(cluster=w115, "POSICION"=w132, "V_VAPOR"=w133) -> (w114:T8)
            n46 = call <vilib>:"Simple Error Handler.vi"("error source (\" \")"=" \"cambioGasesS\" " ("error source (\" \")"), "error in (no error)"=w119) -> ("error out"=w139:errorcluster)  [unwired: 3 in, 4 out]
          }
          frame "cambioGasesF" {
            (unwired) FALSE ("TStable?")
            # "fFlujos: C1: 0.00 C2: 0.00 C3: 0.00 C4: 0.00"
            n47 = Index Array(array=w182, index=w178) -> (element=w169:string)
            n48 = call "Display_Module.vi"("Command"=Display_Command_Control."Generate Event", "error in (no error)"=w180, "Data"="Estableciendo nuevos flujos FLOWBUS" ("element"), "Data Type"=Data_Type."Upd Status") -> ("error out"=w161:errorcluster)  [unwired: 7 in]
            n49 = Scan From String(format string="fFlujos: fC1: %f fC2: %f fC3: %f fC4: %f ", input string=w169) -> (output 1=w173:dbl, output 2=w172:dbl, output 3=w171:dbl, output 4=w170:dbl)  [unwired: 6 in, 3 out]
            n50 = Bundle(w173, w172, w171, w170) -> (w162:cluster{dbl, dbl, dbl, dbl})  [unwired: 1 in]
            n51 = call "_f_bronkhorstWriteAuto.vi"("error in (no error)"=w161, "Datos"=w162) -> ("error out"=w160:errorcluster)  [unwired: 8 in, 1 out]
            n52 = call <vilib>:"Simple Error Handler.vi"("error source (\" \")"=" \"cambioGasesF\" " ("error source (\" \")"), "error in (no error)"=w160) -> ("error out"=w166:errorcluster)  [unwired: 3 in, 4 out]
          }
          frame "cambioValvulas" {
            (unwired) FALSE ("TStable?")
            # "Electrovalvula: ON"
            n53 = Index Array(array=w226, index=w222) -> (element=w201:string)
            n54 = Scan From String(format string="Electrovalvula: %s ", input string=w201) -> (output 1=w206:string)  [unwired: 3 in, 3 out]
            n55 = String Subset(string="", length (rest)=3 ("length (rest)")) -> (substring=w202:string)  [unwired: 1 in]
            n56 = Equal?(x=w206, y="ON") -> (x = y?=w204:bool)
            "Valvula" <- w204
            n57 = Search 1D Array(1D array=string[] ["OFF", "ARR", "ABA", "FRE", "RES"] ("array"), element=w202, start index (0)=0) -> ()  [unwired: 1 out]
            n58 = call "Display_Module.vi"("Command"=Display_Command_Control."Generate Event", "error in (no error)"=w224, "Data"="Estableciendo nueva posicion valvulas" ("element"), "Data Type"=Data_Type."Upd Status") -> ("error out"=w188:errorcluster)  [unwired: 7 in]
            n59 = global read "P2022 TB INCAR GLOBALES.vi" "Arduino"() -> (w185:T5)
            n60 = case shown="0, Default" 0 ("index of element") {
              tunnel: w185 -> [w233 w240 w247 w254 w261]
              tunnel: w204 -> [w232 w239 w246 w253 w260]
              tunnel: [w227 w234 w241 w248 w255] -> w189
              frame 0, Default {
                n61 = Bundle By Name(cluster=w233, "Evalve"=w232, "EVflujo1"=FALSE ("motorUP"), "EVflujo2"=FALSE ("motorDOWN"), "EVflujo3"=FALSE ("motorRST"), "EVflujo4"=FALSE ("motorBRK")) -> (w227:T5)
              }
              frame 1 {
                n62 = Bundle By Name(cluster=w240, "Evalve"=w239, "EVflujo1"=TRUE ("motorUP"), "EVflujo2"=FALSE ("motorDOWN"), "EVflujo3"=FALSE ("motorRST"), "EVflujo4"=FALSE ("motorBRK")) -> (w234:T5)
              }
              frame 2 {
                n63 = Bundle By Name(cluster=w247, "Evalve"=w246, "EVflujo1"=FALSE ("motorUP"), "EVflujo2"=TRUE ("motorDOWN"), "EVflujo3"=FALSE ("motorRST"), "EVflujo4"=FALSE ("motorBRK")) -> (w241:T5)
              }
              frame 3 {
                n64 = Bundle By Name(cluster=w254, "Evalve"=w253, "EVflujo1"=FALSE ("motorUP"), "EVflujo2"=FALSE ("motorDOWN"), "EVflujo3"=FALSE ("motorRST"), "EVflujo4"=TRUE ("motorBRK")) -> (w248:T5)
              }
              frame 4 {
                n65 = Bundle By Name(cluster=w261, "Evalve"=w260, "EVflujo1"=FALSE ("motorUP"), "EVflujo2"=FALSE ("motorDOWN"), "EVflujo3"=TRUE ("motorRST"), "EVflujo4"=FALSE ("motorBRK")) -> (w255:T5)
              }
            }
            "ARDUINO" <- w189
            n66 = Unbundle By Name(w186) -> ("eVal"=w199:bool, "eValPos"=w200:refnum<visa-resource-name>)
            n67 = call "setArduinoMicro.vi"("Enable"=w199, "error in"=w188, "ESTADO"=w189, "VISA resource name"=w200) -> ("error out"=w187:errorcluster, "ESTADO 2"=w192:T5)  [unwired: 6 in]
            n68 = global write "P2022 TB INCAR GLOBALES.vi" "Arduino"(w192) -> ()
            n69 = Unbundle By Name(w192) -> ("EVflujo1"=w197:bool, "EVflujo2"=w196:bool, "EVflujo3"=w195:bool, "EVflujo4"=w194:bool, "Evalve"=w198:bool)
            n70 = call "Time Delay2"("error in (no error)"=w187, "Delay Time (s)"=1.0) -> ("error out"=w212:errorcluster)  [unwired: 9 in]
            n71 = Build Array(w197, w196, w195, w194) -> (w193:bool[])
            n72 = Boolean To (0,1)(Boolean=w198) -> (0, 1=w190:i16)
            n73 = Boolean Array To Number(Boolean array=w193) -> (number=w191:u32)
            n74 = Bundle By Name(cluster=w215, "POSICION"=w191, "V_VAPOR"=w190) -> (w214:T8)
            n75 = call <vilib>:"Simple Error Handler.vi"("error source (\" \")"=" \"cambioValvulas\" " ("error source (\" \")"), "error in (no error)"=w212) -> ("error out"=w211:errorcluster)  [unwired: 3 in, 4 out]
          }
          frame "cambioTemperaturas" {
            w275 = T2 {"Ch1"=0.0, "Ch2"=0.0, "Ch3"=0.0, "Ch4"=0.0} ("NuevoSP")
            w286 = Timing_Module_Control."Initialize Time" ("Command")
            # "Temperatura: SP_S(C): 10.0 r_S(C/min): 0.0 SP_I(C): 11.0 r_I(C/min): 0.0 SP_c(C): 12.0 r_c(C/min): 0.0"
            # "Temperatura: SP_S(C): 10.0 r_S(C/min): 0.0 SP_I(C): 20.0 r_I(C/min): 0.0 SP_c(C): 30.0 r_c(C/min): 0.0"
            n76 = Unbundle By Name(w277) -> ("Eurot"=w278:bool, "Eurothe"=w276:refnum<visa-resource-name>)
            n77 = Index Array(array=w306, index=w302) -> (element=w296:string)
            n78 = call "Display_Module.vi"("Command"=Display_Command_Control."Generate Event", "error in (no error)"=w304, "Data"="Estableciendo nuevas temperaturas" ("element"), "Data Type"=Data_Type."Upd Status") -> ("error out"=w279:errorcluster)  [unwired: 7 in]
            n79 = Scan From String(format string="Temperatura: SP_S(C): %f r_S(C/min): %f SP_I(C): %f r_I(C/min): %f SP_c(C): %f r_c(C/min): %f", input string=w296) -> (output 1=w274:dbl, output 2=w273:dbl, output 3=w272:dbl, output 4=w271:dbl, output 5=w270:dbl, output 6=w269:dbl)  [unwired: 8 in, 3 out]
            n80 = call "Eurotherm_New_Module.vi"("Eurotherm (T:Enable)"=w278, "Command"=Eurotherm_Hardware_Module_Control."Initialize", "error in (no error)"=w279, "VISA resource name"=w276) -> ("error out"=w265:errorcluster)  [unwired: 6 in, 1 out]
            n81 = call "Time Delay11"("error in (no error)"=w265, "Delay Time (s)"=0.125) -> ("error out"=w264:errorcluster)  [unwired: 9 in]
            n82 = Bundle By Name(cluster=w275, "Ch1"=w274, "Ch2"=w272, "Ch3"=w270, "Ch4"=0.0) -> (w263:T2)
            "NuevoSP" <- w263
            n83 = Bundle By Name(cluster=w275, "Ch1"=w273, "Ch2"=w271, "Ch3"=w269, "Ch4"=0.0) -> (w262:T2)
            "RateSP" <- w262
            n84 = call "P116WriteAuto.vi"("error in (no error)"=w264, "NuevoRT"=w262, "NuevoSP"=w263, "Comunicaciones"=w277) -> ("error out"=w281:errorcluster)  [unwired: 5 in, 2 out]
            n85 = call "Eurotherm_New_Module.vi"("Eurotherm (T:Enable)"=w278, "Command"=Eurotherm_Hardware_Module_Control."Shutdown", "error in (no error)"=w281, "VISA resource name"=w276) -> ("error out"=w280:errorcluster)  [unwired: 6 in, 1 out]
            n86 = call "Time Delay7"("error in (no error)"=w280, "Delay Time (s)"=0.05) -> ("error out"=w292:errorcluster)  [unwired: 9 in]
            n87 = call "P2018 Elapsed_Sampling_Seconds_Module.vi"("Command"=w286, "error in (no error)"=w292) -> ("error out"=w290:errorcluster)  [unwired: 7 in, 2 out]
            n88 = call "Elapsed_Step_Minutes_Module.vi"("Command"=w286, "error in (no error)"=w290) -> ("error out"=w285:errorcluster)  [unwired: 7 in, 2 out]
            n89 = local write "MedidaModulo"(u32 0 ("MedidaModulo")) -> ()
            n90 = call "Elapsed_StableT_Minutes_Module.vi"("Command"=w286, "error in (no error)"=w285) -> ("error out"=w284:errorcluster)  [unwired: 7 in, 2 out]
            n91 = call <vilib>:"Simple Error Handler.vi"("error source (\" \")"=" \"cambioTemperaturas\" " ("error source (\" \")"), "error in (no error)"=w284) -> ("error out"=w288:errorcluster)  [unwired: 3 in, 4 out]
          }
          frame "cEstableTemp?" {
            # "Tiempo para estabilizar: Delat_t (s). Ambas temperaturas estarán \ndentro de un margen de Delta_T (C) durante este tiempo\npara considerar que la temperatura es estable."
            # "Maximo tiempo para estabilizar: Max_t (s). \nTranscurrido este tiempo, se considerara estable, \npara no paralizar el programa"
            n92 = Unbundle By Name(w313) -> ("TSET_SUP"=w337:dbl, "TEMP_SUP"=w336:dbl, "TSET_INF"=w335:dbl, "TEMP_INF"=w334:dbl)
            n93 = global read "P2022 TB INCAR GLOBALES.vi" "Delta_T (C)"() -> (w329:dbl)
            n94 = Subtract(x=w337, y=w336) -> (x-y=w333:dbl)
            n95 = Subtract(x=w335, y=w334) -> (x-y=w332:dbl)
            n96 = Absolute Value(x=w333) -> (abs(x)=w331:dbl)
            n97 = Absolute Value(x=w332) -> (abs(x)=w330:dbl)
            n98 = Less?(x=w331, y=w329) -> (x < y?=w327:bool)
            n99 = Less?(x=w330, y=w329) -> (x < y?=w328:bool)
            n100 = And(x=w327, y=w328) -> (x .and. y?=w315:bool)
            n101 = case shown="True" w315 {
              tunnel: w307 -> [w347 w352]
              tunnel: [w346 w351] -> w318
              tunnel: [FALSE ("TStable?") w350] -> w314
              frame False {
                n102 = call "Elapsed_StableT_Minutes_Module.vi"("Command"=Timing_Module_Control."Initialize Time", "error in (no error)"=w347) -> ("error out"=w346:errorcluster)  [unwired: 7 in, 2 out]
              }
              frame True {
                n103 = global read "P2022 TB INCAR GLOBALES.vi" "Delta_t (s)"() -> (w349:dbl)
                n104 = call "Elapsed_StableT_Minutes_Module.vi"("Command"=Timing_Module_Control."Check Time", "error in (no error)"=w352, "Time In"=w349) -> ("error out"=w351:errorcluster, "Time Elapsed"=w350:bool)  [unwired: 6 in, 1 out]
              }
            }
            n105 = global read "P2022 TB INCAR GLOBALES.vi" "Max_t (s)"() -> (w319:dbl)
            n106 = Select(t=", SI", s=w315, f=", NO") -> (s? t:f=w321:string)
            n107 = call "Elapsed_Step_Minutes_Module.vi"("Command"=Timing_Module_Control."Check Time", "error in (no error)"=w318, "Time In"=w319) -> ("error out"=w308:errorcluster, "Elapsed Out"=w310:dbl, "Time Elapsed"=w317:bool)  [unwired: 6 in]
            n108 = Or(x=w314, y=w317) -> (x .or. y?=w316:bool)
            n109 = Number To Fractional String(number=w310, precision (6)=i16 1) -> (F-format string=w324:string)  [unwired: 2 in]
            n110 = Concatenate Strings("Estabilizando, t(s)   ", w324, w321) -> (w309:string)
            n111 = local write "Timestring"(w309) -> ()
            n112 = Select(t=P2018_runAuto_Control."testComando" ("Command"), s=w316, f=P2018_runAuto_Control."cReadTiempo" ("Command")) -> (s? t:f=w338:T11)
            n113 = call <vilib>:"Simple Error Handler.vi"("error source (\" \")"=" \"cEstableTemp?\" " ("error source (\" \")"), "error in (no error)"=w308) -> ("error out"=w311:errorcluster)  [unwired: 3 in, 4 out]
          }
          frame "cReadTiempo" {
            # "Actualiza el tiempo para almacenarlo en fichero de datos"
            n114 = call "P2018 Elapsed_Total_Minutes_Module.vi"("Command"=Timing_Module_Control."Check Time", "error in (no error)"=w367) -> ("error out"=w363:errorcluster, "Elapsed Out"=w355:dbl)  [unwired: 7 in, 1 out]
            n115 = Bundle By Name(cluster=w373, "TIEMPO"=w355) -> (w370:T8)
            n116 = local read "MedidaModulo"() -> (w361:u32)
            n117 = Increment(x=w361) -> (x+1=w360:u32)
            n118 = local write "MedidaModulo"(w360) -> ()
            n119 = local read "Modulo"() -> (w354:u32)
            n120 = call <vilib>:"Simple Error Handler.vi"("error source (\" \")"="\"cReadTiempo\"" ("error source (\" \")"), "error in (no error)"=w363) -> ("error out"=w362:errorcluster)  [unwired: 3 in, 4 out]
            n121 = Greater Or Equal?(x=w360, y=w354) -> (x >= y?=w356:bool)
            n122 = Select(t=P2018_runAuto_Control."cReadGases" ("Command"), s=w356, f=P2018_runAuto_Control."cReadTemperaturas" ("Command")) -> (s? t:f=w357:T11)
          }
          frame "cReadGases" {
            n123 = case shown="True" w403 {
              tunnel: w419 -> [w425 w427]
              tunnel: [w425 w426] -> w417
              frame False {
              }
              frame True {
                n124 = call "Display_Module.vi"("Command"=Display_Command_Control."Generate Event", "error in (no error)"=w427, "Data"="Leyendo flujos de gas", "Data Type"=Data_Type."Upd Status") -> ("error out"=w426:errorcluster)  [unwired: 7 in]
              }
            }
            n125 = call "_s_Bronkhorst Serial Read Flows.vi"("Delay Time (s)"=w404, "Comunicaciones"=w412, "error in (no error)"=w417) -> ("error out"=w383:errorcluster, "Dispositivos"=w381:T4)  [unwired: 7 in]
            n126 = Index Array(array=w381, index (col)=7 ("disabled index (col)")) -> (element=w410:string[])  [unwired: 1 in]
            n127 = Index Array(array=w381, index (col)=6 ("disabled index (col)")) -> (element=w391:string[])  [unwired: 1 in]
            n128 = Fract/Exp String To Number(string=w410) -> (number=w409:dbl[])  [unwired: 3 in, 1 out]
            n129 = Fract/Exp String To Number(string=w391) -> (number=w392:dbl[])  [unwired: 3 in, 1 out]
            n130 = Index Array(array=w409) -> (element #1=w408:dbl, element #2=w407:dbl, element #3=w406:dbl, element #4=w405:dbl)  [unwired: 4 in]
            n131 = Index Array(array=w392) -> (element #1=w393:dbl, element #2=w394:dbl, element #3=w395:dbl, element #4=w379:dbl)  [unwired: 4 in]
            n132 = Bundle By Name(cluster=w418, "sFLUJO1"=w408, "sFLUJO2"=w407, "sFLUJO3"=w406, "sFLUJO4"=w405) -> (w377:T8)
            n133 = Bundle By Name(cluster=w377, "sFSET1"=w393, "sFSET2"=w394, "sFSET3"=w395, "sFSET4"=w379) -> (w376:T8)
            n134 = call "_f_bronkhorstRead.vi"("error in (no error)"=w383) -> ("error out"=w382:errorcluster, "Dispositivos"=w380:T17)  [unwired: 9 in]
            n135 = Index Array(array=w380, index (col)=7 ("disabled index (col)")) -> (element=w397:string[])  [unwired: 1 in]
            n136 = Index Array(array=w380, index (col)=6 ("disabled index (col)")) -> (element=w388:string[])  [unwired: 1 in]
            n137 = Fract/Exp String To Number(string=w397) -> (number=w398:dbl[])  [unwired: 3 in, 1 out]
            n138 = Fract/Exp String To Number(string=w388) -> (number=w387:dbl[])  [unwired: 3 in, 1 out]
            n139 = Index Array(array=w398) -> (element #1=w399:dbl, element #2=w400:dbl, element #3=w401:dbl, element #4=w402:dbl)  [unwired: 4 in]
            n140 = Index Array(array=w387) -> (element #1=w386:dbl, element #2=w385:dbl, element #3=w384:dbl, element #4=w378:dbl)  [unwired: 4 in]
            n141 = Bundle By Name(cluster=w376, "fFLUJO1"=w399, "fFLUJO2"=w400, "fFLUJO3"=w401, "fFLUJO4"=w402) -> (w375:T8)
            n142 = Bundle By Name(cluster=w375, "fFSET1"=w386, "fFSET2"=w385, "fFSET3"=w384, "fFSET4"=w378) -> (w374:T8)
            n143 = local write "MedidaModulo"(u32 0 ("MedidaModulo")) -> ()
            n144 = call <vilib>:"Simple Error Handler.vi"("error source (\" \")"=" \"cReadGases\" " ("error source (\" \")"), "error in (no error)"=w382) -> ("error out"=w414:errorcluster)  [unwired: 3 in, 4 out]
          }
          frame "cReadTemperaturas" {
            w448 = T18 [enum."Add 10", enum."Add 11", enum."Add 12", enum."Add 13"] items=["Add 1", "Add 2", "Add 10", "Add 11", "Add 12", "Add 13"]
            n145 = case shown="True" w431 {
              tunnel: [w462 w467] -> w449
              tunnel: w445 -> [w462 w463]
              frame False {
              }
              frame True {
                n146 = call "Display_Module.vi"("Command"=Display_Command_Control."Generate Event", "error in (no error)"=w463, "Data"="Leyendo temperaturas", "Data Type"=Data_Type."Upd Status") -> ("error out"=w467:errorcluster)  [unwired: 7 in]
              }
            }
            n147 = Unbundle By Name(w444) -> ("Eurot"=w451:bool, "Eurothe"=w450:refnum<visa-resource-name>)
            n148 = call "Eurotherm_New_Module.vi"("Eurotherm (T:Enable)"=w451, "Command"=Eurotherm_Hardware_Module_Control."Initialize", "error in (no error)"=w449, "VISA resource name"=w450) -> ("error out"=w447:errorcluster)  [unwired: 6 in, 1 out]
            n149 = for {
              tunnel: w448 -> [w480] mode=indexing
              tunnel: [w472] -> w440 mode=indexing
              tunnel: [w471] -> w439 mode=indexing
              shift-right: [w469] -> w453
              shift-left: w447 -> [w482]
              tunnel: w451 -> [w479]
              tunnel: [w484] -> _
              shift-right: [w470] -> w452
              shift-left: w450 -> [w470]
              i -> [w478]
              (unwired) 0.125 ("Delay Time (s)")
              w476 = u16 1 items=["0"=1, "1"=10, "2"=100] ("Decimales")
              w477 = u16 1 items=["0"=1, "1"=10, "2"=100] ("Decimales")
              n150 = Equal To 0?(x=w478) -> (x = 0?=w475:bool)
              n151 = Select(t=w477, s=w475, f=w476) -> (s? t:f=w474:u16)
              n152 = call "Eurotherm_New_Module.vi"("Decimales"=w474, "Eurotherm (T:Enable)"=w479, "Command"=Eurotherm_Hardware_Module_Control."Read SP+PV", "error in (no error)"=w482, "Address"=w480, "VISA resource name"=w470) -> ("error out"=w481:errorcluster, "Eurotherm"=w473:T19)  [unwired: 4 in]
              n153 = Number To Decimal String(number=w478) -> (decimal integer string=w485:string)  [unwired: 1 in]
              n154 = Unbundle By Name(w473) -> ("workingSP"=w472:dbl, "processVal"=w471:dbl)
              n155 = call "Time Delay5"("error in (no error)"=w481, "Delay Time (s)"=0.05) -> ("error out"=w469:errorcluster)  [unwired: 9 in]
              n156 = Concatenate Strings("Eurotherm" ("error source (\" \")"), w485) -> (w484:string)
            }
            n157 = VISA Close(VISA resource name=w452, error in (no error)=w453) -> (error out=w443:errorcluster)
            n158 = Index Array(array=w440) -> (element #1=w438:dbl, element #2=w437:dbl, element #3=w436:dbl)  [unwired: 3 in]
            n159 = Index Array(array=w439) -> (element #1=w435:dbl, element #2=w434:dbl, element #3=w433:dbl, element #4=w432:dbl)  [unwired: 4 in]
            n160 = Bundle By Name(cluster=w441, "TSET_SUP"=w438, "TSET_INF"=w437, "TSET_CINTA"=w436, "TEMP_SUP"=w435, "TEMP_INF"=w434, "T_CINTA"=w433, "T_EXTRA"=w432) -> (w442:T8)
            n161 = call <vilib>:"Simple Error Handler.vi"("error source (\" \")"=" \"cReadTemperaturas\" " ("error source (\" \")"), "error in (no error)"=w443) -> ("error out"=w456:errorcluster)  [unwired: 3 in, 4 out]
          }
          frame "cReadTermobalanza" {
            # "Lee siempre termobalanza y guarda datos\nLee y guarda resto 1 de cada 10 veces"
            n162 = case shown="True" w489 {
              tunnel: [w513 w517] -> w503
              tunnel: w501 -> [w513 w514]
              frame False {
              }
              frame True {
                n163 = call "Display_Module.vi"("Command"=Display_Command_Control."Generate Event", "error in (no error)"=w514, "Data"="Leyendo termobalanza", "Data Type"=Data_Type."Upd Status") -> ("error out"=w517:errorcluster)  [unwired: 7 in]
              }
            }
            n164 = Unbundle By Name(w502) -> ("Bal"=w490:bool)
            n165 = call "Multicard III_Hardware_Module.vi"("Multicard (T:Enable)"=w490, "Command"=Multicard_III_Hardware_Module_Control."Read mgr", "error in (no error)"=w503) -> ("error out"=w498:errorcluster, "Output Value"=w504:dbl, "String"=w488:string)  [unwired: 5 in, 1 out]
            n166 = global write "P2022 TB INCAR GLOBALES.vi" "PESO"(w488) -> ()
            n167 = call "Time Delay9"("error in (no error)"=w498, "Delay Time (s)"=0.125) -> ("error out"=w497:errorcluster)  [unwired: 9 in]
            n168 = call "Multicard III_Hardware_Module.vi"("Multicard (T:Enable)"=w490, "Command"=Multicard_III_Hardware_Module_Control."Read T", "error in (no error)"=w497) -> ("error out"=w507:errorcluster, "Output Value"=w508:dbl, "String"=w487:string)  [unwired: 5 in, 1 out]
            n169 = global write "P2022 TB INCAR GLOBALES.vi" "TEMPERATURA"(w487) -> ()
            n170 = case shown="No Error" w507 {
              selector: w507 -> [w519 _]
              tunnel: [w519 errorcluster {"status"=FALSE, "code"=0, "source"=""} ("error out")] -> w492
              tunnel: w504 -> [w521 _]
              tunnel: w499 -> [w523 w524]
              tunnel: [w522 w524] -> w500
              tunnel: w508 -> [w520 _]
              frame No Error {
                n171 = Bundle By Name(cluster=w523, "PESO_TB"=w521, "TEMP_TB"=w520) -> (w522:T8)
              }
              frame Error {
              }
            }
            n172 = call <vilib>:"Simple Error Handler.vi"("error source (\" \")"=" \"cReadTermobalanza\" " ("error source (\" \")"), "error in (no error)"=w492) -> ("error out"=w493:errorcluster)  [unwired: 3 in, 4 out]
          }
          frame "cSaveDatos" {
            n173 = global read "P2022 TB INCAR GLOBALES.vi" "Comments"() -> (w526:string)
            n174 = call "File_Module.vi"("Command"=File_Module_Control."Save Data", "error in (no error)"=w540, "DATOS"=w531, "Comments"=w526) -> ("error out"=w532:errorcluster)  [unwired: 6 in, 1 out]
            n175 = call "Display_Module.vi"("Command"=Display_Command_Control."Generate Event", "error in (no error)"=w532, "Data"=w531, "Data Type"=Data_Type."Update FP") -> ("error out"=w528:errorcluster)  [unwired: 7 in]
            n176 = call <vilib>:"Simple Error Handler.vi"("error source (\" \")"=" \"cSaveDatos\" " ("error source (\" \")"), "error in (no error)"=w528) -> ("error out"=w527:errorcluster)  [unwired: 3 in, 4 out]
          }
          frame "cWait" {
            # "Espera x segundos"
            n177 = global write "P2022 TB INCAR GLOBALES.vi" "Sampling(s)"(w542) -> ()
            n178 = call "P2018 Elapsed_Sampling_Seconds_Module.vi"("Command"=Timing_Module_Control."Check Time", "error in (no error)"=w561, "Time In"=w542) -> ("error out"=w560:errorcluster, "Elapsed Out"=w557:dbl, "Time Elapsed"=w558:bool)  [unwired: 6 in]
            n179 = Subtract(x=w542, y=w557) -> (x-y=w544:dbl)
            n180 = Number To Fractional String(number=w544, precision (6)=i16 1) -> (F-format string=w553:string)  [unwired: 2 in]
            n181 = local read "Timestring"() -> (w543:string)
            n182 = Concatenate Strings(w543, ", Siguiente muestra (s) ", w553) -> (w554:string)
            n183 = call "Display_Module.vi"("Command"=Display_Command_Control."Generate Event", "error in (no error)"=w560, "Data"=w554, "Data Type"=Data_Type."Upd Status") -> ("error out"=w559:errorcluster)  [unwired: 7 in]
            n184 = case shown="True" w558 {
              tunnel: [P2018_runAuto_Control."cWait" ("Command") P2018_runAuto_Control."cEstableTemp?" ("Command")] -> w564
              tunnel: w559 -> [w568 w571]
              tunnel: [w568 w570] -> w550
              frame False {
              }
              frame True {
                n185 = call "P2018 Elapsed_Sampling_Seconds_Module.vi"("Command"=Timing_Module_Control."Initialize Time", "error in (no error)"=w571) -> ("error out"=w570:errorcluster)  [unwired: 7 in, 2 out]
              }
            }
            n186 = call "Time Delay8"("error in (no error)"=w550, "Delay Time (s)"=0.05) -> ("error out"=w546:errorcluster)  [unwired: 9 in]
            n187 = call <vilib>:"Simple Error Handler.vi"("error source (\" \")"=" \"cWait\" " ("error source (\" \")"), "error in (no error)"=w546) -> ("error out"=w545:errorcluster)  [unwired: 3 in, 4 out]
          }
          frame "cambioTiempos" {
            w574 = Timing_Module_Control."Initialize Time" ("Command")
            # "Tiempo de medida (min):  10.0 Frecuencia (seg): 0.0"
            # "Tiempo de medida en segundos"
            # "Tiempo de medida en minutos"
            # "Extrae el tiempo de medida y el de frecuencia de adquisicion"
            n188 = Index Array(array=w591, index=w589) -> (element=w592:string)
            n189 = Scan From String(format string="Tiempo de medida (min): %.1f Frecuencia (seg): %.1f ", input string=w592) -> (output 1=w584:dbl, output 2=w590:dbl)  [unwired: 4 in, 3 out]
            n190 = Multiply(x=w584, y=60.0) -> (x*y=w583:dbl)
            n191 = call "P2018 Elapsed_Sampling_Seconds_Module.vi"("Command"=w574, "error in (no error)"=w582) -> ("error out"=w581:errorcluster)  [unwired: 7 in, 2 out]
            n192 = call "Elapsed_Step_Minutes_Module.vi"("Command"=w574, "error in (no error)"=w581) -> ("error out"=w576:errorcluster)  [unwired: 7 in, 2 out]
            n193 = call "Elapsed_StableT_Minutes_Module.vi"("Command"=w574, "error in (no error)"=w576) -> ("error out"=w575:errorcluster)  [unwired: 7 in, 2 out]
            n194 = local write "MedidaModulo"(u32 0 ("MedidaModulo")) -> ()
            n195 = call <vilib>:"Simple Error Handler.vi"("error source (\" \")"=" \"cambioTiempos\" " ("error source (\" \")"), "error in (no error)"=w575) -> ("error out"=w578:errorcluster)  [unwired: 3 in, 4 out]
          }
          frame "tAgotadoTiempo?" {
            # "Si pulsamos boton SALTAR, finalizamos este paso del programa"
            # "Comprueba si hay que seguir midiendo datos"
            n196 = global read "P2022 TB INCAR GLOBALES.vi" "Pausa"() -> (w602:bool)
            n197 = case shown="True" w602 {
              tunnel: w601 -> [w620 _]
              tunnel: [w620 1000000.0] -> w600
              frame False {
              }
              frame True {
              }
            }
            n198 = call "Elapsed_Step_Minutes_Module.vi"("Command"=Timing_Module_Control."Check Time", "error in (no error)"=w615, "Time In"=w600) -> ("error out"=w594:errorcluster, "Elapsed Out"=w613:dbl, "Time Elapsed"=w614:bool)  [unwired: 6 in]
            n199 = Subtract(x=w600, y=w613) -> (x-y=w607:dbl)
            n200 = Divide(x=w607, y=60.0) -> (x/y=w606:dbl)
            n201 = Number To Fractional String(number=w606, precision (6)=i16 1) -> (F-format string=w610:string)  [unwired: 2 in]
            n202 = global read "P2022 TB INCAR GLOBALES.vi" "Saltar"() -> (w603:bool)
            n203 = Concatenate Strings("Tiempo de medida (min) ", w610) -> (w595:string)
            n204 = Or(x=w614, y=w603) -> (x .or. y?=w604:bool)
            n205 = local write "Timestring"(w595) -> ()
            n206 = case shown="False" w604 {
              tunnel: [P2018_runAuto_Control."tReadTiempo" ("Command") P2018_runAuto_Control."testComando" ("Command")] -> w618
              tunnel: w594 -> [w622 w624]
              tunnel: [w622 w624] -> w596
              frame False {
              }
              frame True {
              }
            }
            n207 = call <vilib>:"Simple Error Handler.vi"("error source (\" \")"=" \"tAgotadoTiempo?\" " ("error source (\" \")"), "error in (no error)"=w596) -> ("error out"=w597:errorcluster)  [unwired: 3 in, 4 out]
          }
          frame "tReadTiempo" {
            # "Solo lee gases y temperaturas una vez de cada \"modulo\" veces\npero la termobalanza la lee siempre"
            # "Actualiza el tiempo para almacenarlo en fichero de datos"
            n208 = call "P2018 Elapsed_Total_Minutes_Module.vi"("Command"=Timing_Module_Control."Check Time", "error in (no error)"=w639) -> ("error out"=w635:errorcluster, "Elapsed Out"=w627:dbl)  [unwired: 7 in, 1 out]
            n209 = Bundle By Name(cluster=w645, "TIEMPO"=w627) -> (w642:T8)
            n210 = local read "MedidaModulo"() -> (w633:u32)
            n211 = Increment(x=w633) -> (x+1=w632:u32)
            n212 = local write "MedidaModulo"(w632) -> ()
            n213 = local read "Modulo"() -> (w626:u32)
            n214 = Greater Or Equal?(x=w632, y=w626) -> (x >= y?=w631:bool)
            n215 = call <vilib>:"Simple Error Handler.vi"("error source (\" \")"="\"tReadTiempo\"" ("error source (\" \")"), "error in (no error)"=w635) -> ("error out"=w634:errorcluster)  [unwired: 3 in, 4 out]
            n216 = Select(t=P2018_runAuto_Control."tReadGases" ("Command"), s=w631, f=P2018_runAuto_Control."tReadTermobalanza" ("Command")) -> (s? t:f=w630:T11)
          }
          frame "tReadGases" {
            n217 = case shown="True" w675 {
              tunnel: [w697 w699] -> w687
              tunnel: w678 -> [w697 w698]
              frame False {
              }
              frame True {
                n218 = call "Display_Module.vi"("Command"=Display_Command_Control."Generate Event", "error in (no error)"=w698, "Data"="Leyendo flujos de gas", "Data Type"=Data_Type."Upd Status") -> ("error out"=w699:errorcluster)  [unwired: 7 in]
              }
            }
            n219 = call "_s_Bronkhorst Serial Read Flows.vi"("Delay Time (s)"=w676, "Comunicaciones"=w679, "error in (no error)"=w687) -> ("error out"=w667:errorcluster, "Dispositivos"=w652:T4)  [unwired: 7 in]
            n220 = Index Array(array=w652, index (col)=7 ("disabled index (col)")) -> (element=w685:string[])  [unwired: 1 in]
            n221 = Index Array(array=w652, index (col)=6 ("disabled index (col)")) -> (element=w661:string[])  [unwired: 1 in]
            n222 = Fract/Exp String To Number(string=w685) -> (number=w684:dbl[])  [unwired: 3 in, 1 out]
            n223 = Fract/Exp String To Number(string=w661) -> (number=w662:dbl[])  [unwired: 3 in, 1 out]
            n224 = Index Array(array=w684) -> (element #1=w683:dbl, element #2=w682:dbl, element #3=w681:dbl, element #4=w680:dbl)  [unwired: 4 in]
            n225 = Index Array(array=w662) -> (element #1=w663:dbl, element #2=w664:dbl, element #3=w665:dbl, element #4=w651:dbl)  [unwired: 4 in]
            n226 = Bundle By Name(cluster=w677, "sFLUJO1"=w683, "sFLUJO2"=w682, "sFLUJO3"=w681, "sFLUJO4"=w680) -> (w649:T8)
            n227 = Bundle By Name(cluster=w649, "sFSET1"=w663, "sFSET2"=w664, "sFSET3"=w665, "sFSET4"=w651) -> (w648:T8)
            n228 = call "_f_bronkhorstRead.vi"("error in (no error)"=w667) -> ("error out"=w666:errorcluster, "Dispositivos"=w653:T17)  [unwired: 9 in]
            n229 = Index Array(array=w653, index (col)=7 ("disabled index (col)")) -> (element=w669:string[])  [unwired: 1 in]
            n230 = Index Array(array=w653, index (col)=6 ("disabled index (col)")) -> (element=w658:string[])  [unwired: 1 in]
            n231 = Fract/Exp String To Number(string=w669) -> (number=w670:dbl[])  [unwired: 3 in, 1 out]
            n232 = Fract/Exp String To Number(string=w658) -> (number=w657:dbl[])  [unwired: 3 in, 1 out]
            n233 = Index Array(array=w670) -> (element #1=w671:dbl, element #2=w672:dbl, element #3=w673:dbl, element #4=w674:dbl)  [unwired: 4 in]
            n234 = Index Array(array=w657) -> (element #1=w656:dbl, element #2=w655:dbl, element #3=w654:dbl, element #4=w650:dbl)  [unwired: 4 in]
            n235 = Bundle By Name(cluster=w648, "fFLUJO1"=w671, "fFLUJO2"=w672, "fFLUJO3"=w673, "fFLUJO4"=w674) -> (w647:T8)
            n236 = Bundle By Name(cluster=w647, "fFSET1"=w656, "fFSET2"=w655, "fFSET3"=w654, "fFSET4"=w650) -> (w646:T8)
            n237 = local write "MedidaModulo"(u32 0 ("MedidaModulo")) -> ()
            n238 = call <vilib>:"Simple Error Handler.vi"("error source (\" \")"=" \"tReadGases\" " ("error source (\" \")"), "error in (no error)"=w666) -> ("error out"=w689:errorcluster)  [unwired: 3 in, 4 out]
          }
          frame "tReadTemperaturas" {
            w721 = T18 [enum."Add 10", enum."Add 11", enum."Add 12", enum."Add 13"] items=["Add 1", "Add 2", "Add 10", "Add 11", "Add 12", "Add 13"]
            n239 = case shown="True" w703 {
              tunnel: [w734 w739] -> w722
              tunnel: w708 -> [w734 w735]
              frame False {
              }
              frame True {
                n240 = call "Display_Module.vi"("Command"=Display_Command_Control."Generate Event", "error in (no error)"=w735, "Data"="Leyendo temperaturas", "Data Type"=Data_Type."Upd Status") -> ("error out"=w739:errorcluster)  [unwired: 7 in]
              }
            }
            n241 = Unbundle By Name(w706) -> ("Eurot"=w724:bool, "Eurothe"=w723:refnum<visa-resource-name>)
            n242 = call "Eurotherm_New_Module.vi"("Eurotherm (T:Enable)"=w724, "Command"=Eurotherm_Hardware_Module_Control."Initialize", "error in (no error)"=w722, "VISA resource name"=w723) -> ("error out"=w720:errorcluster)  [unwired: 6 in, 1 out]
            n243 = for {
              tunnel: w721 -> [w752] mode=indexing
              tunnel: [w744] -> w718 mode=indexing
              tunnel: [w743] -> w717 mode=indexing
              shift-right: [w741] -> w725
              shift-left: w720 -> [w754]
              tunnel: w724 -> [w751]
              tunnel: [w756] -> _
              shift-right: [w742] -> w707
              shift-left: w723 -> [w742]
              i -> [w750]
              (unwired) 0.125 ("Delay Time (s)")
              w748 = u16 1 items=["0"=1, "1"=10, "2"=100] ("Decimales")
              w749 = u16 1 items=["0"=1, "1"=10, "2"=100] ("Decimales")
              n244 = Equal To 0?(x=w750) -> (x = 0?=w747:bool)
              n245 = Select(t=w749, s=w747, f=w748) -> (s? t:f=w746:u16)
              n246 = call "Eurotherm_New_Module.vi"("Decimales"=w746, "Eurotherm (T:Enable)"=w751, "Command"=Eurotherm_Hardware_Module_Control."Read SP+PV", "error in (no error)"=w754, "Address"=w752, "VISA resource name"=w742) -> ("error out"=w753:errorcluster, "Eurotherm"=w745:T19)  [unwired: 4 in]
              n247 = Number To Decimal String(number=w750) -> (decimal integer string=w757:string)  [unwired: 1 in]
              n248 = Unbundle By Name(w745) -> ("workingSP"=w744:dbl, "processVal"=w743:dbl)
              n249 = call "Time Delay10"("error in (no error)"=w753, "Delay Time (s)"=0.05) -> ("error out"=w741:errorcluster)  [unwired: 9 in]
              n250 = Concatenate Strings("Eurotherm" ("error source (\" \")"), w757) -> (w756:string)
            }
            n251 = VISA Close(VISA resource name=w707, error in (no error)=w725) -> (error out=w709:errorcluster)
            n252 = Index Array(array=w718) -> (element #1=w716:dbl, element #2=w715:dbl, element #3=w714:dbl)  [unwired: 3 in]
            n253 = Index Array(array=w717) -> (element #1=w713:dbl, element #2=w712:dbl, element #3=w711:dbl, element #4=w710:dbl)  [unwired: 4 in]
            n254 = Bundle By Name(cluster=w704, "TSET_SUP"=w716, "TSET_INF"=w715, "TSET_CINTA"=w714, "TEMP_SUP"=w713, "TEMP_INF"=w712, "T_CINTA"=w711, "T_EXTRA"=w710) -> (w705:T8)
            n255 = call <vilib>:"Simple Error Handler.vi"("error source (\" \")"=" \"tReadTemperaturas\" " ("error source (\" \")"), "error in (no error)"=w709) -> ("error out"=w728:errorcluster)  [unwired: 3 in, 4 out]
          }
          frame "tReadTermobalanza" {
            # "Lee siempre termobalanza y guarda datos\nLee y guarda resto 1 de cada 10 veces"
            n256 = case shown="True" w761 {
              tunnel: [w785 w789] -> w775
              tunnel: w773 -> [w785 w786]
              frame False {
              }
              frame True {
                n257 = call "Display_Module.vi"("Command"=Display_Command_Control."Generate Event", "error in (no error)"=w786, "Data"="Leyendo termobalanza", "Data Type"=Data_Type."Upd Status") -> ("error out"=w789:errorcluster)  [unwired: 7 in]
              }
            }
            n258 = Unbundle By Name(w774) -> ("Bal"=w762:bool)
            n259 = call "Multicard III_Hardware_Module.vi"("Multicard (T:Enable)"=w762, "Command"=Multicard_III_Hardware_Module_Control."Read mgr", "error in (no error)"=w775) -> ("error out"=w770:errorcluster, "Output Value"=w776:dbl, "String"=w759:string)  [unwired: 5 in, 1 out]
            n260 = global write "P2022 TB INCAR GLOBALES.vi" "PESO"(w759) -> ()
            n261 = call "Time Delay3"("error in (no error)"=w770, "Delay Time (s)"=0.125) -> ("error out"=w769:errorcluster)  [unwired: 9 in]
            n262 = call "Multicard III_Hardware_Module.vi"("Multicard (T:Enable)"=w762, "Command"=Multicard_III_Hardware_Module_Control."Read T", "error in (no error)"=w769) -> ("error out"=w779:errorcluster, "Output Value"=w780:dbl, "String"=w760:string)  [unwired: 5 in, 1 out]
            n263 = global write "P2022 TB INCAR GLOBALES.vi" "TEMPERATURA"(w760) -> ()
            n264 = case shown="No Error" w779 {
              selector: w779 -> [w791 _]
              tunnel: [w791 errorcluster {"status"=FALSE, "code"=0, "source"=""} ("error out")] -> w764
              tunnel: w776 -> [w793 _]
              tunnel: w771 -> [w795 w796]
              tunnel: [w794 w796] -> w772
              tunnel: w780 -> [w792 _]
              frame No Error {
                n265 = Bundle By Name(cluster=w795, "PESO_TB"=w793, "TEMP_TB"=w792) -> (w794:T8)
              }
              frame Error {
              }
            }
            n266 = call <vilib>:"Simple Error Handler.vi"("error source (\" \")"=" \"tReadTermobalanza\" " ("error source (\" \")"), "error in (no error)"=w764) -> ("error out"=w765:errorcluster)  [unwired: 3 in, 4 out]
          }
          frame "tSaveDatos" {
            n267 = global read "P2022 TB INCAR GLOBALES.vi" "Comments"() -> (w798:string)
            n268 = call "File_Module.vi"("Command"=File_Module_Control."Save Data", "error in (no error)"=w812, "DATOS"=w803, "Comments"=w798) -> ("error out"=w804:errorcluster)  [unwired: 6 in, 1 out]
            n269 = call "Display_Module.vi"("Command"=Display_Command_Control."Generate Event", "error in (no error)"=w804, "Data"=w803, "Data Type"=Data_Type."Update FP") -> ("error out"=w800:errorcluster)  [unwired: 7 in]
            n270 = call <vilib>:"Simple Error Handler.vi"("error source (\" \")"=" \"tSaveDatos\" " ("error source (\" \")"), "error in (no error)"=w800) -> ("error out"=w799:errorcluster)  [unwired: 3 in, 4 out]
          }
          frame "tWait" {
            # "Espera x segundos"
            n271 = global write "P2022 TB INCAR GLOBALES.vi" "Sampling(s)"(w814) -> ()
            n272 = call "P2018 Elapsed_Sampling_Seconds_Module.vi"("Command"=Timing_Module_Control."Check Time", "error in (no error)"=w835, "Time In"=w814) -> ("error out"=w834:errorcluster, "Elapsed Out"=w831:dbl, "Time Elapsed"=w832:bool)  [unwired: 6 in]
            n273 = Subtract(x=w814, y=w831) -> (x-y=w823:dbl)
            n274 = Divide(x=w823, y=1.0) -> (x/y=w822:dbl)
            n275 = Number To Fractional String(number=w822, precision (6)=i16 1) -> (F-format string=w827:string)  [unwired: 2 in]
            n276 = local read "Timestring"() -> (w819:string)
            n277 = Concatenate Strings(w819, "; Siguiente muestra (s) ", w827) -> (w828:string)
            n278 = call "Display_Module.vi"("Command"=Display_Command_Control."Generate Event", "error in (no error)"=w834, "Data"=w828, "Data Type"=Data_Type."Upd Status") -> ("error out"=w833:errorcluster)  [unwired: 7 in]
            n279 = case shown="True" w832 {
              tunnel: [P2018_runAuto_Control."tWait" ("Command") P2018_runAuto_Control."tAgotadoTiempo?" ("Command")] -> w838
              tunnel: w833 -> [w842 w845]
              tunnel: [w842 w844] -> w821
              frame False {
              }
              frame True {
                n280 = call "P2018 Elapsed_Sampling_Seconds_Module.vi"("Command"=Timing_Module_Control."Initialize Time", "error in (no error)"=w845) -> ("error out"=w844:errorcluster)  [unwired: 7 in, 2 out]
              }
            }
            n281 = call "Time Delay6"("error in (no error)"=w821, "Delay Time (s)"=0.05) -> ("error out"=w816:errorcluster)  [unwired: 9 in]
            n282 = call <vilib>:"Simple Error Handler.vi"("error source (\" \")"=" \"tWait\" " ("error source (\" \")"), "error in (no error)"=w816) -> ("error out"=w815:errorcluster)  [unwired: 3 in, 4 out]
          }
          frame "finalizar" {
            n283 = call "Display_Module.vi"("Command"=Display_Command_Control."Generate Event", "error in (no error)"=w859, "Data"="Fin de programa", "Data Type"=Data_Type."Upd Status") -> ("error out"=w854:errorcluster)  [unwired: 7 in]
            n284 = call "Display_Module.vi"("Command"=Display_Command_Control."Generate Event", "error in (no error)"=w854, "Data"=0, "Data Type"=Data_Type."En/Dis FP Ctls") -> ("error out"=w849:errorcluster)  [unwired: 7 in]
            n285 = call <vilib>:"Simple Error Handler.vi"("error source (\" \")"=" \"finalizar\" " ("error source (\" \")"), "error in (no error)"=w849) -> ("error out"=w848:errorcluster)  [unwired: 3 in, 4 out]
          }
        }
        "Datos" <- w32
        "TStable" <- w29
        n286 = call "P2018 TB INCAR_Stop.vi"("error in (no error)"=w44, "Stop"=enum16{"Continue", "Stop", "Default"}."Default") -> ("error out"=w45:errorcluster, "Stop?"=w43:bool)  [unwired: 8 in]
        n287 = global write "P2022 TB INCAR GLOBALES.vi" "TStable?"(w29) -> ()
        n288 = Or(x=w43, y=w48) -> (x .or. y?=w49:bool)
        n289 = Wait (ms)(milliseconds to wait=u32 10) -> ()  [unwired: 1 out]
      }
      "Modulo" <- "ModuloIN"
    }
    frame Error {
    }
  }
  n290 = call "Display_Module.vi"("Command"=Display_Command_Control."Generate Event", "error in (no error)"=w7, "Data"="Fin de programa", "Data Type"=Data_Type."Upd Status") -> ("error out"=w14:errorcluster)  [unwired: 7 in]
  n291 = call "Display_Module.vi"("Command"=Display_Command_Control."Generate Event", "error in (no error)"=w14, "Data"=0, "Data Type"=Data_Type."En/Dis FP Ctls") -> ("error out"=w5:errorcluster)  [unwired: 7 in]
  n292 = call "P2018 TB INCAR_Stop.vi"("error in (no error)"=w5, "Stop"=enum16{"Continue", "Stop", "Default"}."Continue") -> ("error out"=→"error out":errorcluster)  [unwired: 8 in, 1 out]
